vi "KHE - Main.vi"() -> ()   [LabVIEW 2016]
doc: "Use this template to build a producer/consumer design pattern with events to produce queue items. Use this design pattern instead of the User Interface Event Handler pattern for user interfaces when you want to execute code asynchronously in response to an event without slowing the user interface responsiveness."
uses:
  Hall Effect Library/Public/Controls/Resisitivity.ctl
  Hall Effect Library/Public/Controls/Magnets.ctl
  Hall Effect Library/Public/Controls/Ammeters.ctl
  Hall Effect Library/Public/Controls/I-Sources.ctl
  Hall Effect Library/Public/Controls/Switches.ctl
  Hall Effect Library/Public/Controls/Voltmeters.ctl
  <vilib>/Utility/miscctls.llb/LVPointTypeDef.ctl
  Hall Effect Library/Public/Communication/Decode Message Data (Status).vi
  Hall Effect Library/Public/Communication/Decode Message Data (New Data).vi
  Hall Effect Library/Public/Communication/Decode Message Data (Test End).vi
  Hall Effect Library/Hall Effect Library.lvlib
panel:
  in  "Front Panel Window Default Size":T1={"Horizontal"=980, "Vertical"=600}
  in  "cmdSaveData":bool
  in  "cmdClearData":bool
  out "Test Progress":u8(slide) scale=0.0..100.0
  in  "Instrument Locations":T2
  in  "Instruments":T8={"Magnet"=enum."Manual", "Ammeter"=enum."648X", "Current Source"=enum."622X", "Switch"=enum."3706A", "Voltmeter"=enum."2182A"}
  in  "Special Guard Parameters":T9={"Low to Earth"=enum."Off", "Inner Shield"=enum."Cable Guard"}
  out "Test In Progress":bool
  in  "cmdStop":bool
  in  "cmdStart":bool
  out "Status":string
  out "Programable Event":refnum<user-event>
  in  "Tab Control":T10(tab)
  in  "Test Type":T11
  in  "Test Identification":T12
  in  "Test Input Parameters":T14={"Current Level "=0.001, "Compliance Level"=1.0, "Soak Time"=0.0, "NPLC Voltmeter"=1.0, "Count Voltmeter"=1, "NPLC Ammeter"=1.0, "Count Ammeter"=1, "Sample Resistivity"=enum."Low", "Sample Thickness"=1.0, "Magnetic Flux"=0.57, "Units"=enum."T", "Sample Dimensions x"=1.0, "Sample Dimensions y"=1.0, "Sample Dimensions D1"=1.0, "Sample Dimensions D2"=1.0, "Sample Width Ws"=1.0, "Slot Number of 3765 Card"=1} {"Slot Number of 3765 Card" min=1 max=6 step=1; "NPLC Ammeter" min=0.01 max=10.0; "NPLC Voltmeter" min=0.01 max=10.0 format="%^#_6g"; "Count Ammeter" min=1 max=1024; "Count Voltmeter" min=1 max=1024; "Magnetic Flux" min=0.0; "Soak Time" min=0.0 format="%^#_6g"; "Sample Thickness" min=0.0; "Current Level" min=0.0 max=0.1 format="%^#_6e"; "Compliance Level" min=0.0 max=8.0 format="%^#_6g"}
  out "Test Date":string
  out "Hall Effect Results":T15 {"µH" format="%^#_6e"; "RHD" format="%^#_6e"; "RHC" format="%^#_6e"; "RHAvg" format="%^#_6e"; "n/p" format="%^#_6e"}
  out "Van Der Pauw Resistance Results":T16 {"PAvg" format="%^#_6e"; "PB" format="%^#_6e"; "PA" format="%^#_6e"; "QB" format="%^#_6e"; "QA" format="%^#_6e"; "fA" format="%^#_6e"; "fB" format="%^#_6e"}
  out "Hall Measurements":T17 {"V4" format="%^#_6e"; "V8" format="%^#_6e"; "V7" format="%^#_6e"; "V3" format="%^#_6e"; "V2" format="%^#_6e"; "V6" format="%^#_6e"; "V5" format="%^#_6e"; "V1" format="%^#_6e"}
  out "Van Der Pauw Measurements":T17 {"V7" format="%^#_6e"; "V8" format="%^#_6e"; "V6" format="%^#_6e"; "V5" format="%^#_6e"; "V4" format="%^#_6e"; "V3" format="%^#_6e"; "V2" format="%^#_6e"; "V1" format="%^#_6e"}
  out "Test Settings":T18={"Current Level"=0.0, "Compliance Level"=0.0, "Soak Time"=0.0, "NPLC Voltmeter"=1.0, "Count Voltmeter"=1, "NPLC Ammeter"=1.0, "Count Ammeter"=1, "Sample Resistivity"=enum."Low", "Sample Thickness"=0.0, "Magnetic Flux"=0.0, "Units"=enum."T", "Sample Dimensions x"=0.0, "Sample Dimension y"=0.0, "Sample Dimensions D1"=0.0, "Sample Dimensions D2"=0.0, "Sample Width Ws"=0.0, "Slot Number of 3765 Card"=0} {"NPLC Ammeter" min=0.01 max=10.0; "NPLC Voltmeter" min=0.01 max=10.0 format="%^#_6g"; "Count Ammeter" min=1 max=1024; "Count Voltmeter" min=1 max=1024; "Soak Time" format="%^#_6g"; "Compliance Level" format="%^#_6g"; "Current Level" format="%^#_6e"}
  out "Sample Name":string
  out "User Name":string
  out "8-Contact Sample Results":T19 {"uH" format="%^#_6e"; "RAVG" format="%^#_6e"; "PB" format="%^#_6e"; "PA" format="%^#_6e"; "Pavg" format="%^#_6e"}
  out "6-Contact Sample Results":T20 {"uH" format="%^#_6e"; "RH2" format="%^#_6e"; "RH1" format="%^#_6e"; "RAVG" format="%^#_6e"; "PB" format="%^#_6e"; "PA" format="%^#_6e"; "Pavg" format="%^#_6e"}
  out "8-Contact Sample Hall Voltage Measurements":cluster{"V1":dbl, "V2":dbl, "V3":dbl, "V4":dbl} {"V4" format="%^#_6e"; "V3" format="%^#_6e"; "V2" format="%^#_6e"; "V1" format="%^#_6e"}
  out "6-Contact Sample Hall Voltage Measurements":T21 {"V4" format="%^#_6e"; "V8" format="%^#_6e"; "V7" format="%^#_6e"; "V6" format="%^#_6e"; "V5" format="%^#_6e"; "V3" format="%^#_6e"; "V2" format="%^#_6e"; "V1" format="%^#_6e"}
  out "Bar Sample Results":T22 {"Hall Mobility" format="%^#_6e"; "n/p" format="%^#_6e"; "Resitivity" format="%^#_6e"}
  out "8-Contact Sample Resitivity Measurements":cluster{"V1":dbl, "V2":dbl, "V3":dbl, "V4":dbl} {"V4" format="%^#_6e"; "V3" format="%^#_6e"; "V2" format="%^#_6e"; "V1" format="%^#_6e"}
  out "6-Contact Sample Resitivity Measurements":cluster{"V1":dbl, "V2":dbl, "V3":dbl, "V4":dbl} {"V4" format="%^#_6e"; "V3" format="%^#_6e"; "V2" format="%^#_6e"; "V1" format="%^#_6e"}
  out "Bar Sample Measurements":T23 {"Hall Voltage" format="%^#_6e"; "Voltage Resistivity" format="%^#_6e"}
  in  "cmdBack":bool
  in  "cmdIndex":bool
  in  "Help Browser":refnum<k7>(container)
  # "Selecting Resistivity"
  # "Source Settings"
  # "A"
  # "V"
  # "s"
  # "Measure Settings"
  # "Ammeter"
  # "Voltmeter"
  # "Other Settings"
  # "cm"
  # "cm"
  # "cm"
  # "cm"
  # "cm"
  # "cm"
  # "Hall Coefficient"
  # "cm^3/C"
  # "cm^2/V s"
  # "cm^-3"
  # "cm^3/C"
  # "cm^3/C"
  # "Geometric Factor"
  # "Resistance Ratio"
  # "Resistivity"
  # "Ohm cm"
  # "Ohm cm"
  # "Ohm cm"
  # "Magnet"
  # "Pos"
  # "Volts"
  # "Neg"
  # "Polarity"
  # "Volts"
  # "A"
  # "V"
  # "s"
  # "NPLC"
  # "cm"
  # "Measure Count"
  # "cm"
  # "cm"
  # "cm"
  # "cm"
  # "cm"
  # "Resistivity"
  # "Hall Coefficient"
  # "Hall Mobility"
  # "PAvg"
  # "RH"
  # "µH"
  # "Ohm cm"
  # "cm^3/C"
  # "cm^2/V s"
  # "PA"
  # "Ohm cm"
  # "PB"
  # "Ohm cm"
  # "Resistivity"
  # "Hall Coefficient"
  # "Hall Mobility"
  # "PAvg"
  # "µH"
  # "RAvg"
  # "Ohm cm"
  # "cm^3/C"
  # "cm^2/V s"
  # "PA"
  # "RH1"
  # "Ohm cm"
  # "cm^3/C"
  # "PB"
  # "RH2"
  # "Ohm cm"
  # "cm^3/C"
  # "Magnet"
  # "V1"
  # "V2"
  # "Pos"
  # "Volts"
  # "Neg"
  # "Polarity"
  # "V3"
  # "V4"
  # "V1"
  # "V2"
  # "V5"
  # "V6"
  # "Magnet"
  # "Pos"
  # "Volts"
  # "Neg"
  # "Polarity"
  # "V3"
  # "V4"
  # "V7"
  # "V8"
  # "p"
  # "µH"
  # "Ohm cm"
  # "cm^-3"
  # "cm^2/V s"
  # "V1"
  # "V2"
  # "Current"
  # "Pos"
  # "Volts"
  # "Neg"
  # "Direction"
  # "V3"
  # "V4"
  # "V1"
  # "V2"
  # "Current"
  # "Pos"
  # "Volts"
  # "Neg"
  # "Direction"
  # "V3"
  # "V4"
  # "Vr"
  # "Vh"
  # "Volts"
  # "Volts"
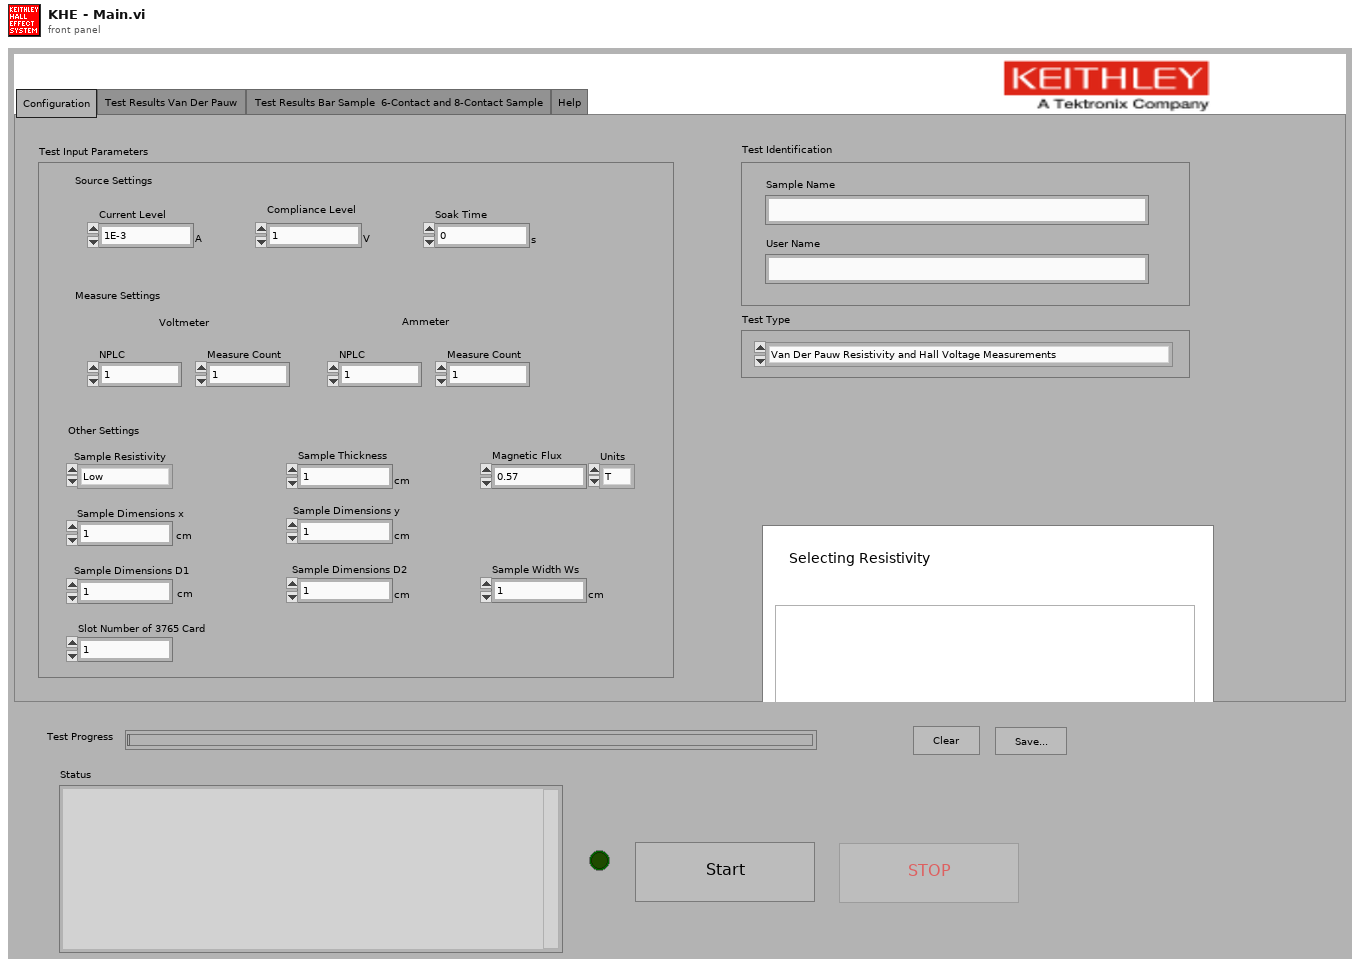
[diagram p1: front panel]
types:
  T1 = typedef "LVPointTypeDef.ctl" = cluster{"Horizontal":i16, "Vertical":i16}
  T2 = cluster{"Magnet Location":refnum<visa-resource-name>, "Ammeter Location":refnum<visa-resource-name>, "Current Source Location":refnum<visa-resource-name>, "Switch Location":refnum<visa-resource-name>, "Voltmeter Location":refnum<visa-resource-name>}
  T3 = typedef "Hall Effect Library.lvlib/Magnets.ctl" = enum16{"Manual"}
  T4 = typedef "Hall Effect Library.lvlib/Ammeters.ctl" = enum16{"None", "648X"}
  T5 = typedef "Hall Effect Library.lvlib/I-Sources.ctl" = enum16{"622X", "26XX"}
  T6 = typedef "Hall Effect Library.lvlib/Switches.ctl" = enum16{"3706A"}
  T7 = typedef "Hall Effect Library.lvlib/Voltmeters.ctl" = enum16{"2000", "2182A", "3706A"}
  T8 = cluster{"Magnet":T3, "Ammeter":T4, "Current Source":T5, "Switch":T6, "Voltmeter":T7}
  T9 = cluster{"Low to Earth":enum16{"On", "Off"}, "Inner Shield":enum16{"Output Lo ", "Cable Guard"}}
  T10 = enum32{"Configuration", "Test Results Van Der Pauw ", "Test Results Bar Sample  6-Contact and 8-Contact Sample ", "Help"}
  T11 = cluster{"Test Type":enum16{"Van Der Pauw Resistivity and Hall Voltage Measurements", "Bar Sample Resistivity and Hall Voltage Measurement", "6-Contact Sample Resistivity and Hall Voltage Measurement", "8-Contact Sample Resistivity and Hall Voltage Measurement"}}
  T12 = cluster{"Sample Name":string, "User Name":string}
  T13 = typedef "Hall Effect Library.lvlib/Resisitivity.ctl" = enum16{"Low", "High"}
  T14 = cluster{"Current Level ":dbl, "Compliance Level":dbl, "Soak Time":dbl, "NPLC Voltmeter":dbl, "Count Voltmeter":i32, "NPLC Ammeter":dbl, "Count Ammeter":i32, "Sample Resistivity":T13, "Sample Thickness":dbl, "Magnetic Flux":dbl, "Units":enum16{"Gs", "T"}, "Sample Dimensions x":dbl, "Sample Dimensions y":dbl, "Sample Dimensions D1":dbl, "Sample Dimensions D2":dbl, "Sample Width Ws":dbl, "Slot Number of 3765 Card":u32}
  T15 = cluster{"RHD":dbl, "RHC":dbl, "RHAvg":dbl, "µH":dbl, "n/p":dbl}
  T16 = cluster{"fA":dbl, "fB":dbl, "QA":dbl, "QB":dbl, "PAvg":dbl, "PA":dbl, "PB":dbl}
  T17 = cluster{"V1":dbl, "V2":dbl, "V3":dbl, "V4":dbl, "V5":dbl, "V6":dbl, "V7":dbl, "V8":dbl}
  T18 = cluster{"Current Level":dbl, "Compliance Level":dbl, "Soak Time":dbl, "NPLC Voltmeter":dbl, "Count Voltmeter":i32, "NPLC Ammeter":dbl, "Count Ammeter":i32, "Sample Resistivity":T13, "Sample Thickness":dbl, "Magnetic Flux":dbl, "Units":enum16{"Gs", "T"}, "Sample Dimensions x":dbl, "Sample Dimension y":dbl, "Sample Dimensions D1":dbl, "Sample Dimensions D2":dbl, "Sample Width Ws":dbl, "Slot Number of 3765 Card":u8}
  T19 = cluster{"Pavg":dbl, "PA":dbl, "PB":dbl, "RAVG":dbl, "uH":dbl}
  T20 = cluster{"Pavg":dbl, "PA":dbl, "PB":dbl, "RAVG":dbl, "RH1":dbl, "RH2":dbl, "uH":dbl}
  T21 = cluster{"V1":dbl, "V2":dbl, "V3":dbl, "V5":dbl, "V6":dbl, "V7":dbl, "V8":dbl, "V4":dbl}
  T22 = cluster{"Resitivity":dbl, "n/p":dbl, "Hall Mobility":dbl}
  T23 = cluster{"Voltage Resistivity":dbl, "Hall Voltage":dbl}
  T24 = cluster{"Test Identification":cluster{"Sample Name":string, "User Name":string}, "Test Input Parameters":cluster{"Current Level ":dbl, "Compliance Level":dbl, "Soak Time":dbl, "NPLC Voltmeter":dbl, "Count Voltmeter":i32, "NPLC Ammeter":dbl, "Count Ammeter":i32, "Sample Resistivity":T13, "Sample Thickness":dbl, "Magnetic Flux":dbl, "Units":enum16{"Gs", "T"}, "Sample Dimensions x":dbl, "Sample Dimensions y":dbl, "Sample Dimensions D1":dbl, "Sample Dimensions D2":dbl, "Sample Width Ws":dbl, "Slot Number of 3765 Card":u32}, "Test Type":cluster{"Test Type":enum16{"Van Der Pauw Resistivity and Hall Voltage Measurements", "Bar Sample Resistivity and Hall Voltage Measurement", "6-Contact Sample Resistivity and Hall Voltage Measurement", "8-Contact Sample Resistivity and Hall Voltage Measurement"}}}
  T25 = enum16{"open", "replace", "create", "open or create", "replace or create", "replace or create with confirmation"}
  T26 = enum32{"invalid app kind", "Development System", "Run Time System", "Student Edition", "Embedded LabVIEW", "Evaluation", "Custom"}
  T27 = typedef "LVAllMonitorsDisplayTypeDef.ctl" = cluster{"Bounds":cluster{"Left":i16, "Top":i16, "Right":i16, "Bottom":i16}, "Depth":i16}[]
  T28 = cluster{"Bounds":cluster{"Left":i16, "Top":i16, "Right":i16, "Bottom":i16}, "Depth":i16}
  T29 = cluster{"Left":i16, "Top":i16, "Right":i16, "Bottom":i16}
  T30 = typedef "LVRectTypeDef.ctl" = cluster{"Left":i16, "Top":i16, "Right":i16, "Bottom":i16}
  T31 = enum16{"Van Der Pauw Resistivity and Hall Voltage Measurements", "Bar Sample Resistivity and Hall Voltage Measurement", "6-Contact Sample Resistivity and Hall Voltage Measurement", "8-Contact Sample Resistivity and Hall Voltage Measurement"}
  T32 = typedef "Hall Effect Library.lvlib/Message Types.ctl" = enum16{"Status", "New Data", "Test End Normal", "Test End User Abort", "Test End Error"}
  T33 = typedef "Hall Effect Library.lvlib/Data Items.ctl" = enum16{"V1 Van Der Pauw", "V2 Van Der Pauw", "V3 Van Der Pauw", "V4 Van Der Pauw", "V5 Van Der Pauw", "V6 Van Der Pauw", "V7 Van Der Pauw", "V8 Van Der Pauw", "V1 Hall Effect", "V2 Hall Effect", "V3 Hall Effect", "V4 Hall Effect", "V5 Hall Effect", "V6  Hall Effect", "V7 Hall Effect", "V8 Hall Effect", "V1 Res Bar", "V1 Hall Bar", "V1 Res 6-Cot", "V2 Res 6-Cot", "V3 Res 6-Cot", "V4 Res 6-Cot", "V1 Hall 6-Cot", "V2 Hall 6-Cot", "V3 Hall 6-Cot", "V4 Hall 6-Cot", "V5 Hall 6-Cot", "V6 Hall 6-Cot", "V7 Hall 6-Cot", "V8 Hall 6-Cot", "V1 Res 8-Cot", "V2 Res 8-Cot", "V3 Res 8-Cot", "V4 Res 8-Cot", "V1 Hall 8-Cot", "V2 Hall 8-Cot", "V3 Hall 8-Cot", "V4 Hall 8-Cot", "Van Der Pauw Results", "Hall Effect Results", "Bar Sample Resistivity Results", "Bar Sample Hall Results", "6-Contact Resistivity Results", "6-Contact Hall Results", "8-Contact Resistivity Results", "8-Contact Hall Results"}
  T34 = cluster{"Van Der Pauw Voltages[0]":dbl, "Van Der Pauw Voltages[1]":dbl, "Van Der Pauw Voltages[2]":dbl, "Van Der Pauw Voltages[3]":dbl, "Van Der Pauw Voltages[4]":dbl, "Van Der Pauw Voltages[5]":dbl, "Van Der Pauw Voltages[6]":dbl, "Van Der Pauw Voltages[7]":dbl}
  T35 = cluster{"Hall Effect Voltages[0]":dbl, "Hall Effect Voltages[1]":dbl, "Hall Effect Voltages[2]":dbl, "Hall Effect Voltages[3]":dbl, "Hall Effect Voltages[4]":dbl, "Hall Effect Voltages[5]":dbl, "Hall Effect Voltages[6]":dbl, "Hall Effect Voltages[7]":dbl}
  T36 = cluster{"6-Contact Sample Resistivity Voltage[0]":dbl, "6-Contact Sample Resistivity Voltage[1]":dbl, "6-Contact Sample Resistivity Voltage[2]":dbl, "6-Contact Sample Resistivity Voltage[3]":dbl}
  T37 = cluster{"6-Contact Sample Hall Voltages[0]":dbl, "6-Contact Sample Hall Voltages[1]":dbl, "6-Contact Sample Hall Voltages[2]":dbl, "6-Contact Sample Hall Voltages[3]":dbl, "6-Contact Sample Hall Voltages[4]":dbl, "6-Contact Sample Hall Voltages[5]":dbl, "6-Contact Sample Hall Voltages[6]":dbl, "6-Contact Sample Hall Voltages[7]":dbl}
  T38 = cluster{"8-Contact Sample Resistivity Voltages[0]":dbl, "8-Contact Sample Resistivity Voltages[1]":dbl, "8-Contact Sample Resistivity Voltages[2]":dbl, "8-Contact Sample Resistivity Voltages[3]":dbl}
  T39 = cluster{"8-Contact Sample Hall Voltages[0]":dbl, "8-Contact Sample Hall Voltages[1]":dbl, "8-Contact Sample Hall Voltages[2]":dbl, "8-Contact Sample Hall Voltages[3]":dbl}
  T40 = cluster{"fA":dbl, "fB":dbl, "QA":dbl, "QB":dbl, "pAvg":dbl, "pA":dbl, "pB":dbl}
  T41 = cluster{"RHD":dbl, "RHC":dbl, "RHAvg":dbl, "uH":dbl, "n/p":dbl}
  T42 = cluster{"RAvg":dbl, "RH1":dbl, "RH2":dbl, "uH":dbl}
  T43 = typedef "Hall Effect Library.lvlib/Tests.ctl" = enum16{"Van Der Pauw", "Hall Effect", "Bar Sample Resistivity", "Bar Sample Hall ", "6-Contact Sample Resistivity", "6-Contact Sample Hall", "8-Contact Sample Resistivity", "8-Contact Sample Hall", ""}
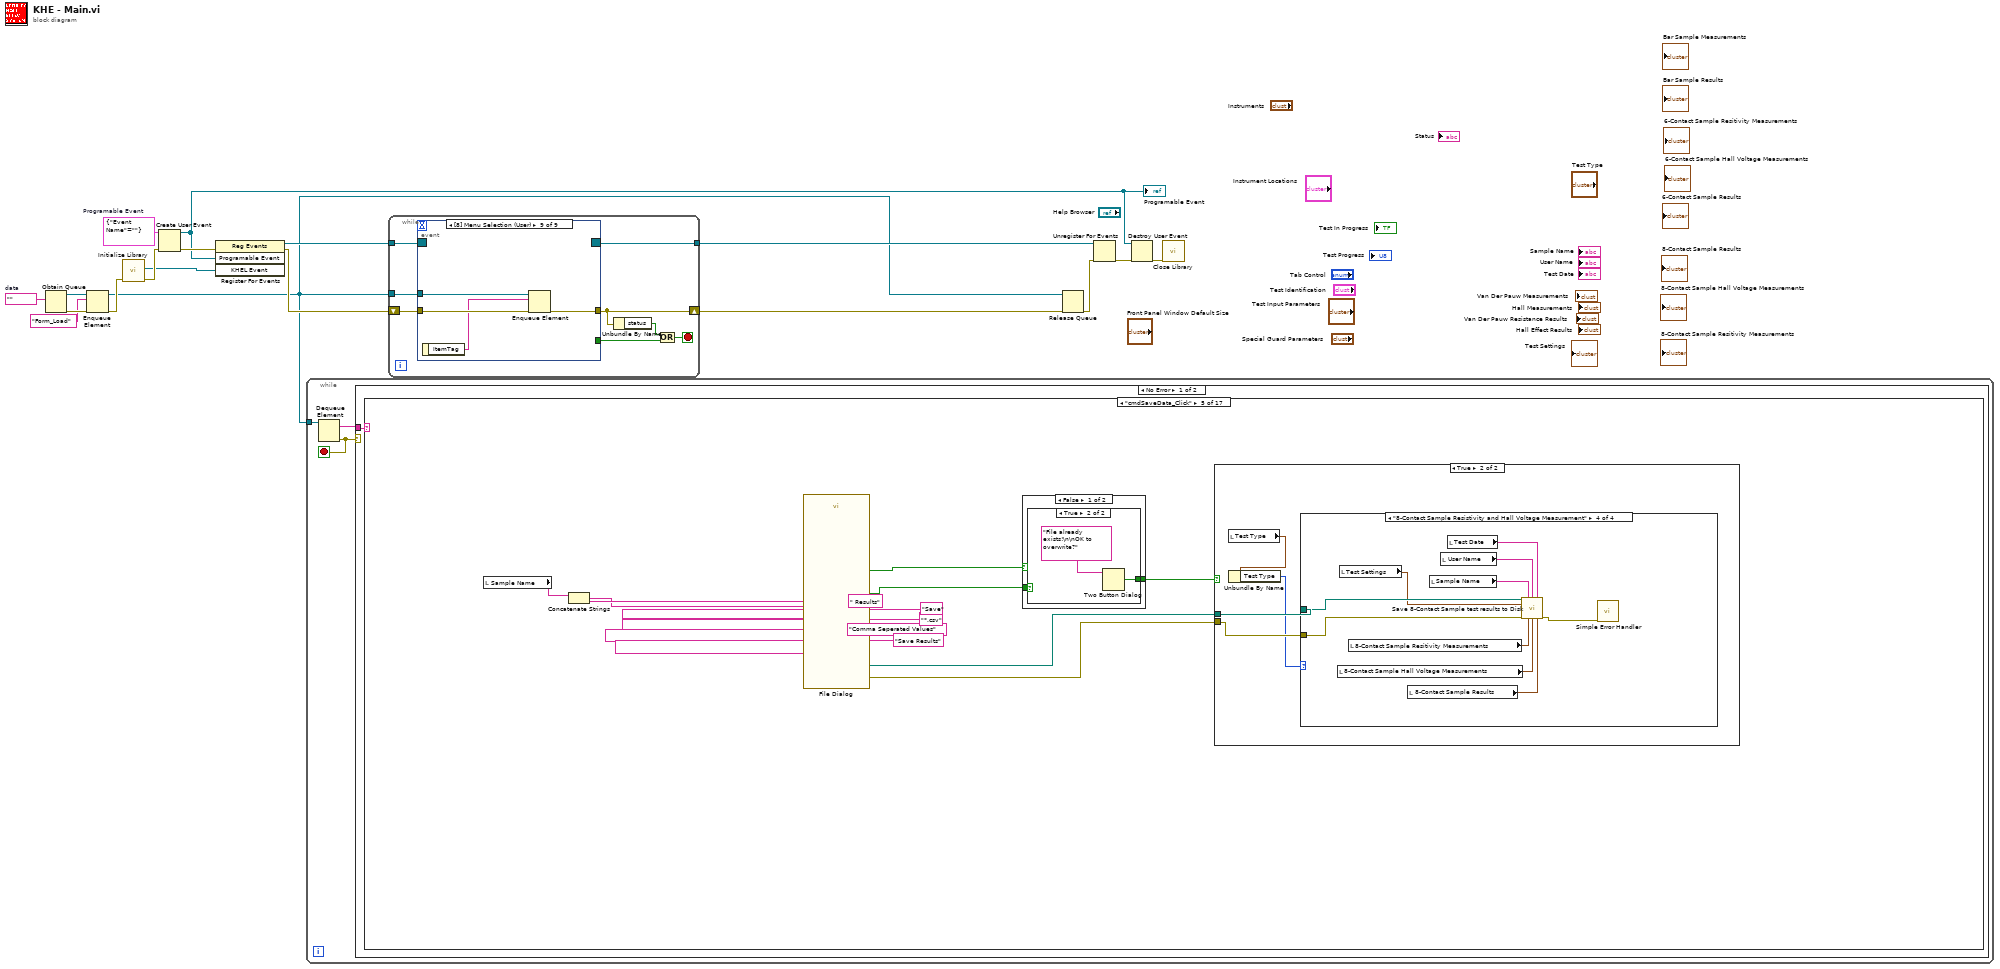
[diagram p0: block diagram]
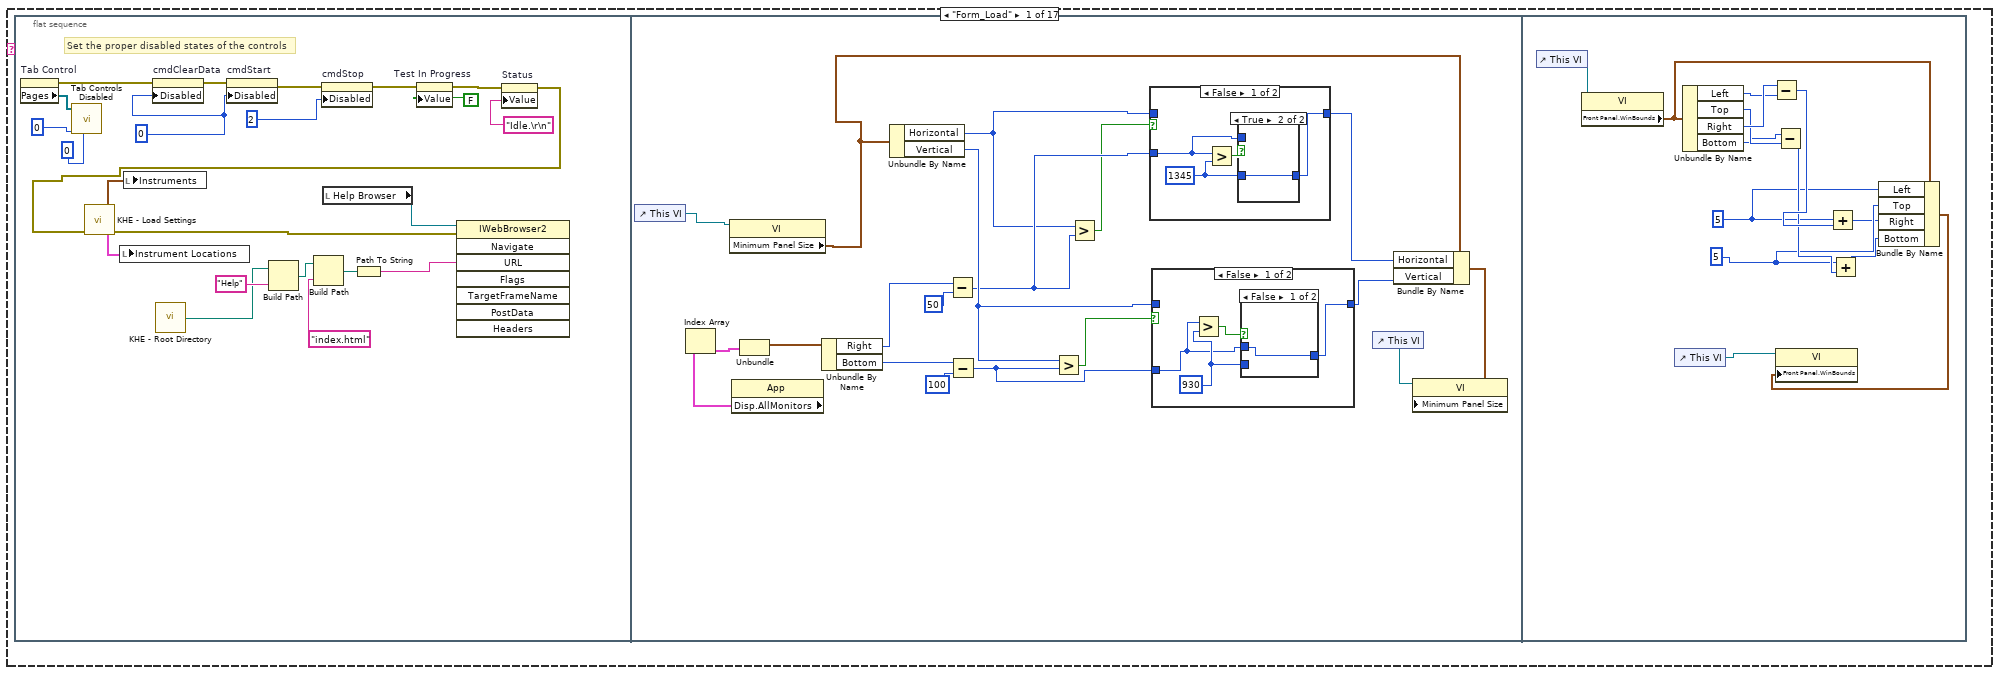
[diagram p2: hidden frame]
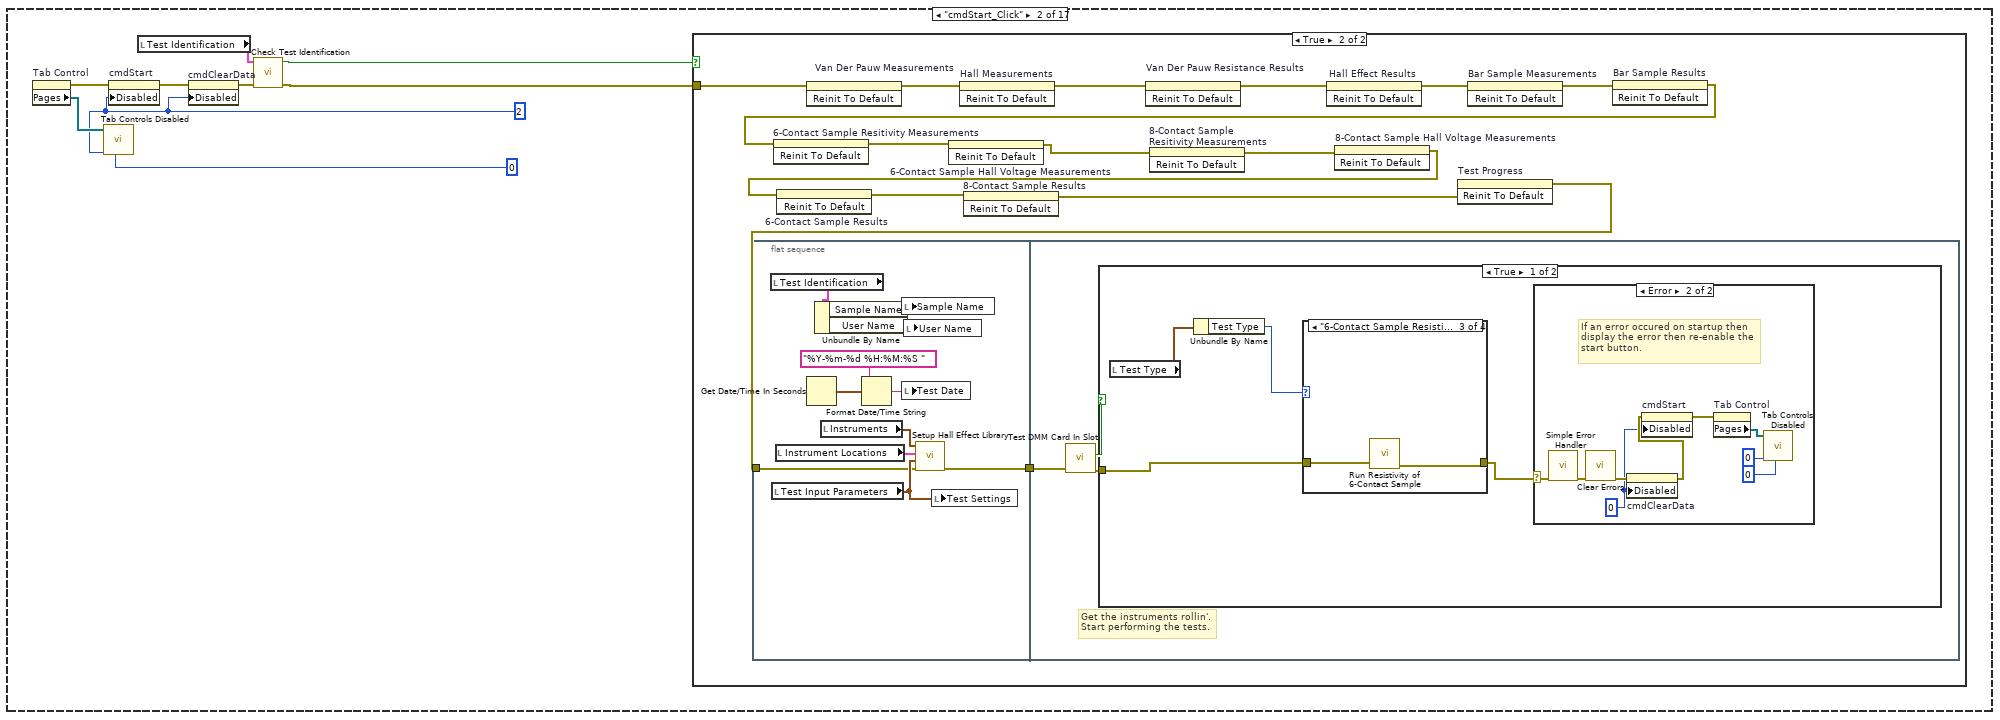
[diagram p7: hidden frame]
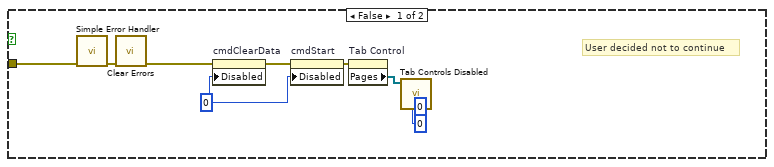
[diagram p8: hidden frame]
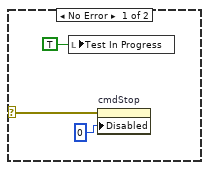
[diagram p9: hidden frame]
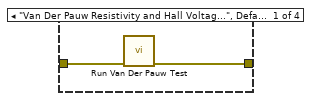
[diagram p10: hidden frame]
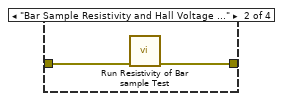
[diagram p11: hidden frame]
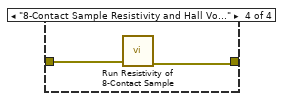
[diagram p12: hidden frame]
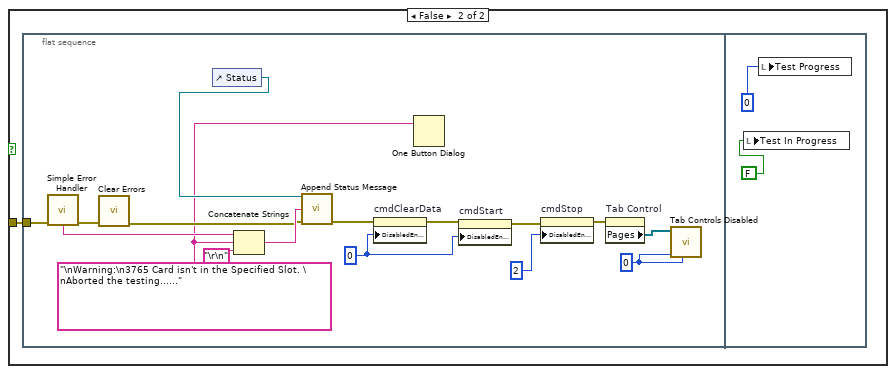
[diagram p13: hidden frame]
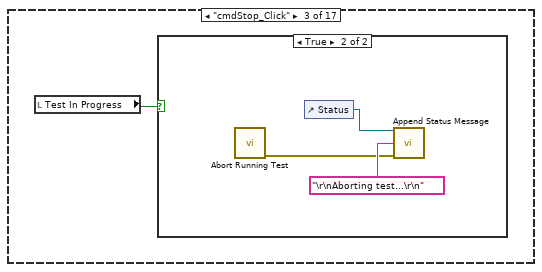
[diagram p14: hidden frame]
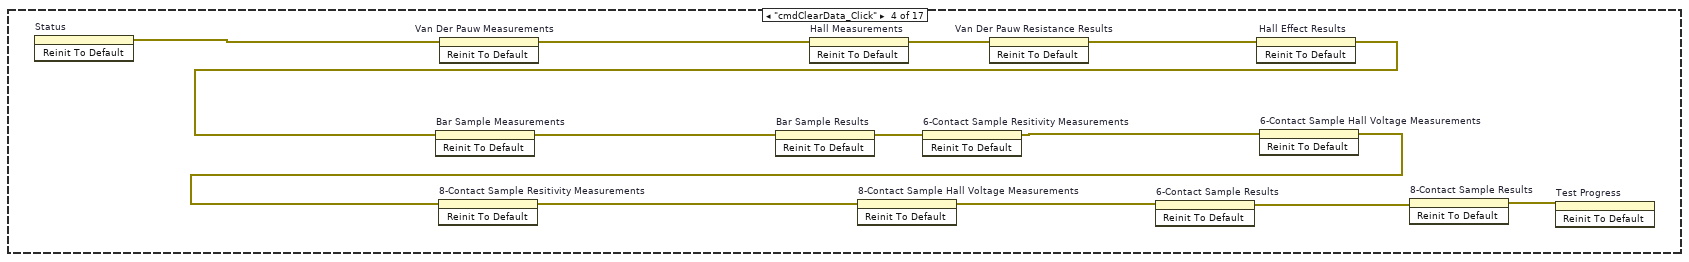
[diagram p16: hidden frame]
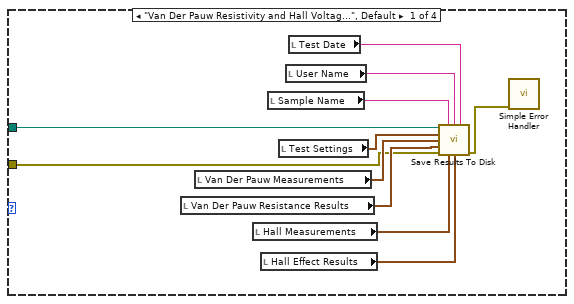
[diagram p18: hidden frame]
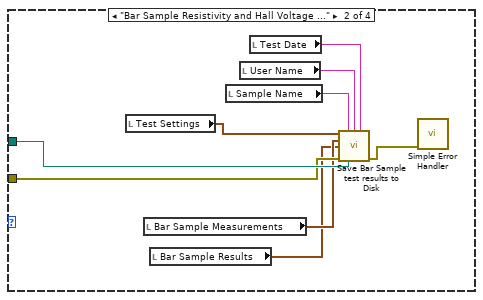
[diagram p19: hidden frame]
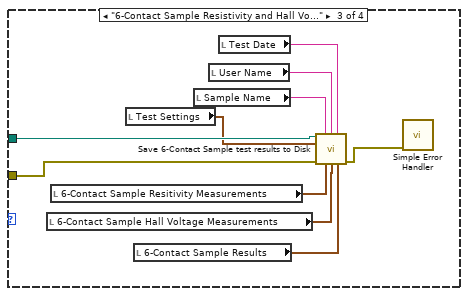
[diagram p20: hidden frame]
diagram:
  w16 = cluster{"Event Name":string} {"Event Name"=""}  # Programable Event
  w17 = ""  # data
  n1 = Obtain Queue(element data type=w17) -> (queue out=w9:refnum<queue>, error out=w8:errorcluster)  [unwired: 3 in, 2 out]
  n2 = Enqueue Element(queue=w9, element="Form_Load", error in (no error)=w8) -> (queue out=w2:refnum<queue>, error out=w6:errorcluster)  [unwired: 2 out]
  n3 = call "Initialize Library.vi"("error in (no error)"=w6) -> ("error out"=w5:errorcluster, "KHEL Event"=w3:refnum<user-event>)  [unwired: 9 out]
  n4 = Create User Event(user event datatype=w16, error in=w5) -> (user event=w4:refnum<user-event>, error out=w15:errorcluster)
  "Programable Event" <- w4
  n5 = register-events(error in=w15, w4, w3) -> (reference out=w10:refnum<event-registration>, error out=w14:errorcluster)  [unwired: 1 in]
  n6 = while {
    tunnel: w2 -> [w21]
    stop <- w20 stop-if-true
    n7 = Dequeue Element(queue=w21) -> (element=w19:string, error out=w20:errorcluster)  [unwired: 1 in, 3 out]
    n8 = case shown="No Error" w20 {
      tunnel: w19 -> [w22 _]
      frame No Error {
        n9 = case shown="\"cmdSaveData_Click\"" w22 {
          frame "Form_Load" {
            n10 = flat-sequence {
              frame #0 {
                w25 = u8 0 ("Disabled")
                # "Set the proper disabled states of the controls"
                n11 = property on="Tab Control" class="TabCtl (strict)"() -> (error out=w32:errorcluster, "Pages"=w44:refnum<vi>[])  [unwired: 2 in, 1 out]
                n12 = call "Tab Controls Disabled.vi"("Page"=0, "Disabled"=u8 0, "Tab Control Pages"=w44) -> ()  [unwired: 9 out]
                n13 = property on="cmdClearData" class="Bool"(error in=w32, "Disabled"=w25) -> (error out=w33:errorcluster)  [unwired: 1 in, 1 out]
                n14 = call "KHE - Root Directory.vi"() -> ("Project Root Directory"=w28:path)  [unwired: 1 out]
                n15 = property on="cmdStart" class="Bool"(error in=w33, "Disabled"=w25) -> (error out=w45:errorcluster)  [unwired: 1 in, 1 out]
                n16 = Build Path(base path=w28, name or relative path="Help") -> (appended path=w37:path)
                n17 = Build Path(base path=w37, name or relative path="index.html") -> (appended path=w35:path)
                n18 = property on="cmdStop" class="Bool"(error in=w45, "Disabled"=u8 2) -> (error out=w43:errorcluster)  [unwired: 1 in, 1 out]
                n19 = local read "Help Browser"() -> (w39:refnum<k7>)
                n20 = Path To String(path=w35) -> (string=w34:string)
                n21 = property on="Test In Progress" class="Bool (strict)"(error in=w43, "Value"=FALSE ("Test In Progress")) -> (error out=w41:errorcluster)  [unwired: 1 in, 1 out]
                n22 = property on="Status" class="Str"(error in=w41, "Value"="Idle.\r\n" ("Status")) -> (error out=w23:errorcluster)  [unwired: 1 in, 1 out]
                n23 = call "KHE - Load Settings.vi"("error in (no error)"=w23) -> ("error out"=w29:errorcluster, "Instrument Locations"=w31:T2, "Instruments"=w30:T8)  [unwired: 8 out]
                n24 = local write "Instrument Locations"(w31) -> ()
                n25 = local write "Instruments"(w30) -> ()
                n26 = invoke class="IWebBrowser2" method="Navigate"(reference=w39, error in=w29, "URL"=w34) -> ()  [unwired: 5 in, 8 out]
              }
              frame #1 {
                n27 = control-ref of="This VI"() -> (w46:refnum<vi>)
                n28 = property class="VI"(reference=w46) -> ("Minimum Panel Size"=w64:T1)  [unwired: 1 in, 2 out]
                n29 = property class="App"() -> ("Disp.AllMonitors"=w47:T27)  [unwired: 2 in, 2 out]
                n30 = Index Array(array=w47) -> (element=w48:T28)  [unwired: 1 in]
                n31 = Unbundle(w48) -> ("Bounds"=w49:T29)  [unwired: 1 out]
                n32 = Unbundle By Name(w49) -> ("Right"=w50:i16, "Bottom"=w52:i16)
                n33 = Unbundle By Name(w64) -> ("Horizontal"=w56:i16, "Vertical"=w58:i16)
                n34 = Subtract(x=w50, y=50) -> (x-y=w57:i32)
                n35 = Subtract(x=w52, y=100) -> (x-y=w59:i32)
                n36 = Greater?(x=w58, y=w59) -> (0:w55:bool)
                n37 = Greater?(x=w56, y=w57) -> (0:w54:bool)
                n38 = case shown="False" w54 {
                  tunnel: w56 -> [_ w78]
                  tunnel: w57 -> [w72 _]
                  tunnel: [w73 w78] -> w60
                  frame False {
                    w74 = 1345
                    n39 = Greater?(x=w72, y=w74) -> (0:w75:bool)
                    n40 = case shown="True" w75 {
                      tunnel: w74 -> [_ w77]
                      tunnel: [w76 w77] -> w73
                      tunnel: w72 -> [w76 _]
                      frame False {
                      }
                      frame True {
                      }
                    }
                  }
                  frame True {
                  }
                }
                n41 = case shown="False" w55 {
                  tunnel: w58 -> [_ w71]
                  tunnel: w59 -> [w65 _]
                  tunnel: [w66 w71] -> w61
                  frame False {
                    w67 = 930
                    n42 = Greater?(x=w65, y=w67) -> (0:w68:bool)
                    n43 = case shown="False" w68 {
                      tunnel: w67 -> [_ w70]
                      tunnel: [w69 w70] -> w66
                      tunnel: w65 -> [w69 _]
                      frame False {
                      }
                      frame True {
                      }
                    }
                  }
                  frame True {
                  }
                }
                n44 = control-ref of="This VI"() -> (w63:refnum<vi>)
                n45 = Bundle By Name(cluster=w64, "Horizontal"=w60, "Vertical"=w61) -> (w62:T1)
                n46 = property class="VI"(reference=w63, "Minimum Panel Size"=w62) -> ()  [unwired: 1 in, 2 out]
              }
              frame #2 {
                w84 = 5
                w85 = 5
                n47 = control-ref of="This VI"() -> (w92:refnum<vi>)
                n48 = property class="VI"(reference=w92) -> ("Front Panel.WinBounds"=w79:T30)  [unwired: 1 in, 2 out]
                n49 = control-ref of="This VI"() -> (w81:refnum<vi>)
                n50 = Unbundle By Name(w79) -> ("Left"=w90:i16, "Top"=w89:i16, "Right"=w91:i16, "Bottom"=w88:i16)
                n51 = Subtract(x=w91, y=w90) -> (x-y=w87:i16)
                n52 = Subtract(x=w88, y=w89) -> (x-y=w86:i16)
                n53 = Add(x=w85, y=w87) -> (x+y=w83:i32)
                n54 = Add(x=w84, y=w86) -> (x+y=w82:i32)
                n55 = Bundle By Name(cluster=w79, "Left"=w85, "Top"=w84, "Right"=w83, "Bottom"=w82) -> (w80:T30)
                n56 = property class="VI"(reference=w81, "Front Panel.WinBounds"=w80) -> ()  [unwired: 1 in, 2 out]
              }
            }
          }
          frame "cmdStart_Click" {
            w93 = u8 2 ("Disabled")
            n57 = property on="Tab Control" class="TabCtl (strict)"() -> (error out=w101:errorcluster, "Pages"=w100:refnum<vi>[])  [unwired: 2 in, 1 out]
            n58 = call "Tab Controls Disabled.vi"("Page"=0, "Disabled"=w93, "Tab Control Pages"=w100) -> ()  [unwired: 9 out]
            n59 = property on="cmdStart" class="Bool"(error in=w101, "Disabled"=w93) -> (error out=w95:errorcluster)  [unwired: 1 in, 1 out]
            n60 = local read "Test Identification"() -> (w98:T12)
            n61 = property on="cmdClearData" class="Bool"(error in=w95, "Disabled"=w93) -> (error out=w94:errorcluster)  [unwired: 1 in, 1 out]
            n62 = call "Check Test Identification.vi"("error in (no error)"=w94, "Test Identification"=w98) -> ("error out"=w97:errorcluster, "Continue?"=w96:bool)  [unwired: 8 out]
            n63 = case shown="True" w96 {
              tunnel: w97 -> [w105 w121]
              frame False {
                w102 = u8 0 ("Disabled")
                # "User decided not to continue"
                n64 = call <vilib>:"Simple Error Handler.vi"("error in (no error)"=w105) -> ("error out"=w110:errorcluster)  [unwired: 1 in, 7 out]
                n65 = call <vilib>:"Clear Errors.vi"("error in (no error)"=w110) -> ("error out"=w103:errorcluster)  [unwired: 1 in, 5 out]
                n66 = property on="cmdClearData" class="Bool"(error in=w103, "Disabled"=w102) -> (error out=w104:errorcluster)  [unwired: 1 in, 1 out]
                n67 = property on="cmdStart" class="Bool"(error in=w104, "Disabled"=w102) -> (error out=w108:errorcluster)  [unwired: 1 in, 1 out]
                n68 = property on="Tab Control" class="TabCtl (strict)"(error in=w108) -> ("Pages"=w109:refnum<vi>[])  [unwired: 1 in, 2 out]
                n69 = call "Tab Controls Disabled.vi"("Page"=0, "Disabled"=u8 0, "Tab Control Pages"=w109) -> ()  [unwired: 9 out]
              }
              frame True {
                n70 = flat-sequence {
                  tunnel: w122 -> [w127]
                  tunnel: [w126] -> w120
                  tunnel: w120 -> [w139]
                  frame #0 {
                    n71 = local read "Test Identification"() -> (w131:T12)
                    n72 = local read "Test Input Parameters"() -> (w130:T14)
                    n73 = local read "Instrument Locations"() -> (w128:T2)
                    n74 = Get Date/Time In Seconds() -> (seconds since 1Jan1904=w134:timestamp)
                    n75 = Unbundle By Name(w131) -> ("Sample Name"=w133:string, "User Name"=w132:string)
                    n76 = local read "Instruments"() -> (w129:T8)
                    n77 = Format Date/Time String(time format string (%c)="%Y-%m-%d %H:%M:%S ", seconds (now)=w134) -> (date/time string=w135:string)  [unwired: 1 out]
                    n78 = local write "Sample Name"(w133) -> ()
                    n79 = local write "Test Date"(w135) -> ()
                    n80 = local write "User Name"(w132) -> ()
                    n81 = call "Setup Hall Effect Library.vi"("error in (no error)"=w127, "Test Input Parameters"=w130, "Instrument Locations"=w128, "Instruments"=w129) -> ("error out"=w126:errorcluster)  [unwired: 7 out]
                    n82 = local write "Test Settings"(w130) -> ()
                  }
                  frame #1 {
                    # "Get the instruments rollin'.\nStart performing the tests."
                    n83 = call "Test DMM Card In Slot.vi"("error in (no error)"=w139) -> ("error out"=w137:errorcluster, "In Card Flag"=w138:bool)  [unwired: 9 in]
                    n84 = case shown="True" w138 {
                      tunnel: w137 -> [w143 w164]
                      frame True {
                        n85 = local read "Test Type"() -> (w141:T11)
                        n86 = Unbundle By Name(w141) -> ("Test Type"=w140:T31)
                        n87 = case shown="\"6-Contact Sample Resistivity and Hall Voltage Measurement\"" w140 {
                          tunnel: w143 -> [w156 w159 w161 w163]
                          tunnel: [w157 w158 w160 w162] -> w142
                          frame "Van Der Pauw Resistivity and Hall Voltage Measurements", Default {
                            n88 = call "Run Van Der Pauw Test.vi"("error in (no error)"=w156) -> ("error out"=w157:errorcluster)  [unwired: 10 out]
                          }
                          frame "Bar Sample Resistivity and Hall Voltage Measurement" {
                            n89 = call "Run Resistivity of Bar sample Test.vi"("error in (no error)"=w159) -> ("error out"=w158:errorcluster)  [unwired: 10 in]
                          }
                          frame "6-Contact Sample Resistivity and Hall Voltage Measurement" {
                            n90 = call "Run Resistivity of 6-Contact Sample.vi"("error in (no error)"=w161) -> ("error out"=w160:errorcluster)  [unwired: 10 in]
                          }
                          frame "8-Contact Sample Resistivity and Hall Voltage Measurement" {
                            n91 = call "Run Resistivity of 8-Contact Sample.vi"("error in (no error)"=w163) -> ("error out"=w162:errorcluster)  [unwired: 10 in]
                          }
                        }
                        n92 = case shown="Error" w142 {
                          selector: w142 -> [w145 w155]
                          frame No Error {
                            n93 = local write "Test In Progress"(TRUE ("Test In Progress")) -> ()
                            n94 = property on="cmdStop" class="Bool"(error in=w145, "Disabled"=u8 0) -> ()  [unwired: 1 in, 2 out]
                          }
                          frame Error {
                            w147 = u8 0 ("Disabled")
                            # "If an error occured on startup then\ndisplay the error then re-enable the\nstart button."
                            n95 = call <vilib>:"Simple Error Handler.vi"("error in (no error)"=w155) -> ("error out"=w154:errorcluster)  [unwired: 1 in, 7 out]
                            n96 = call <vilib>:"Clear Errors.vi"("error in (no error)"=w154) -> ("error out"=w149:errorcluster)  [unwired: 1 in, 5 out]
                            n97 = property on="cmdClearData" class="Bool"(error in=w149, "Disabled"=w147) -> (error out=w148:errorcluster)  [unwired: 1 in, 1 out]
                            n98 = property on="cmdStart" class="Bool"(error in=w148, "Disabled"=w147) -> (error out=w152:errorcluster)  [unwired: 1 in, 1 out]
                            n99 = property on="Tab Control" class="TabCtl (strict)"(error in=w152) -> ("Pages"=w153:refnum<vi>[])  [unwired: 1 in, 2 out]
                            n100 = call "Tab Controls Disabled.vi"("Page"=0, "Disabled"=u8 0, "Tab Control Pages"=w153) -> ()  [unwired: 9 out]
                          }
                        }
                      }
                      frame False {
                        n101 = flat-sequence {
                          tunnel: w164 -> [w179]
                          frame #0 {
                            w166 = 0
                            w170 = 0
                            w165 = "\nWarning:\n3765 Card isn't in the Specified Slot. \nAborted the testing......"
                            n102 = call <vilib>:"Simple Error Handler.vi"("error in (no error)"=w179) -> ("error out"=w175:errorcluster, "message"=w177:string)  [unwired: 1 in, 6 out]
                            n103 = call <vilib>:"Clear Errors.vi"("error in (no error)"=w175) -> ("error out"=w174:errorcluster)  [unwired: 1 in, 5 out]
                            n104 = control-ref of="Status"() -> (w180:refnum<vi>)
                            n105 = Concatenate Strings(w177, w165, "\r\n") -> (w176:string)
                            n106 = call "Append Status Message.vi"("Str Refnum"=w180, "Message"=w176, "error in (no error)"=w174) -> ("error out"=w173:errorcluster)  [unwired: 12 in]
                            n107 = property on="cmdClearData" class="Bool"(error in=w173, "DisabledEnum"=w170) -> (error out=w172:errorcluster)  [unwired: 1 in, 1 out]
                            n108 = One Button Dialog(message=w165) -> ()  [unwired: 1 in, 1 out]
                            n109 = property on="cmdStart" class="Bool"(error in=w172, "DisabledEnum"=w170) -> (error out=w171:errorcluster)  [unwired: 1 in, 1 out]
                            n110 = property on="cmdStop" class="Bool"(error in=w171, "DisabledEnum"=2) -> (error out=w168:errorcluster)  [unwired: 1 in, 1 out]
                            n111 = property on="Tab Control" class="TabCtl (strict)"(error in=w168) -> ("Pages"=w167:refnum<vi>[])  [unwired: 1 in, 2 out]
                            n112 = call "Tab Controls Disabled.vi"("Page"=w166, "Disabled"=w166, "Tab Control Pages"=w167) -> ()  [unwired: 9 in]
                          }
                          frame #1 {
                            n113 = local write "Test In Progress"(FALSE) -> ()
                            n114 = local write "Test Progress"(0) -> ()
                          }
                        }
                      }
                    }
                  }
                }
                n115 = invoke on="Van Der Pauw Measurements" class="Clust (strict)" method="Reinit To Default"(error in=w121) -> (error out=w125:errorcluster)  [unwired: 2 in, 2 out]
                n116 = invoke on="Hall Measurements" class="Clust (strict)" method="Reinit To Default"(error in=w125) -> (error out=w124:errorcluster)  [unwired: 2 in, 2 out]
                n117 = invoke on="Van Der Pauw Resistance Results" class="Clust (strict)" method="Reinit To Default"(error in=w124) -> (error out=w123:errorcluster)  [unwired: 2 in, 2 out]
                n118 = invoke on="Hall Effect Results" class="Clust (strict)" method="Reinit To Default"(error in=w123) -> (error out=w119:errorcluster)  [unwired: 2 in, 2 out]
                n119 = invoke on="Bar Sample Measurements" class="Clust (strict)" method="Reinit To Default"(error in=w119) -> (error out=w118:errorcluster)  [unwired: 2 in, 2 out]
                n120 = invoke on="Bar Sample Results" class="Clust (strict)" method="Reinit To Default"(error in=w118) -> (error out=w117:errorcluster)  [unwired: 2 in, 2 out]
                n121 = invoke on="6-Contact Sample Resitivity Measurements" class="Clust (strict)" method="Reinit To Default"(error in=w117) -> (error out=w116:errorcluster)  [unwired: 2 in, 2 out]
                n122 = invoke on="6-Contact Sample Hall Voltage Measurements" class="Clust (strict)" method="Reinit To Default"(error in=w116) -> (error out=w115:errorcluster)  [unwired: 2 in, 2 out]
                n123 = invoke on="8-Contact Sample Resitivity Measurements" class="Clust (strict)" method="Reinit To Default"(error in=w115) -> (error out=w114:errorcluster)  [unwired: 2 in, 2 out]
                n124 = invoke on="8-Contact Sample Hall Voltage Measurements" class="Clust (strict)" method="Reinit To Default"(error in=w114) -> (error out=w113:errorcluster)  [unwired: 2 in, 2 out]
                n125 = invoke on="6-Contact Sample Results" class="Clust (strict)" method="Reinit To Default"(error in=w113) -> (error out=w112:errorcluster)  [unwired: 2 in, 2 out]
                n126 = invoke on="8-Contact Sample Results" class="Clust (strict)" method="Reinit To Default"(error in=w112) -> (error out=w111:errorcluster)  [unwired: 2 in, 2 out]
                n127 = invoke on="Test Progress" class="Slide (strict)" method="Reinit To Default"(error in=w111) -> (error out=w122:errorcluster)  [unwired: 2 in, 2 out]
              }
            }
          }
          frame "cmdStop_Click" {
            n128 = local read "Test In Progress"() -> (w183:bool)
            n129 = case shown="True" w183 {
              frame False {
              }
              frame True {
                n130 = call "Abort Running Test.vi"() -> ("error out"=w184:errorcluster)  [unwired: 1 in, 10 out]
                n131 = control-ref of="Status"() -> (w186:refnum<vi>)
                n132 = call "Append Status Message.vi"("Str Refnum"=w186, "Message"="\r\nAborting test...\r\n", "error in (no error)"=w184) -> ()  [unwired: 13 out]
              }
            }
          }
          frame "cmdClearData_Click" {
            n133 = invoke on="Status" class="Str" method="Reinit To Default"() -> (error out=w187:errorcluster)  [unwired: 3 in, 2 out]
            n134 = invoke on="Van Der Pauw Measurements" class="Clust (strict)" method="Reinit To Default"(error in=w187) -> (error out=w199:errorcluster)  [unwired: 2 in, 2 out]
            n135 = invoke on="Hall Measurements" class="Clust (strict)" method="Reinit To Default"(error in=w199) -> (error out=w198:errorcluster)  [unwired: 2 in, 2 out]
            n136 = invoke on="Van Der Pauw Resistance Results" class="Clust (strict)" method="Reinit To Default"(error in=w198) -> (error out=w197:errorcluster)  [unwired: 2 in, 2 out]
            n137 = invoke on="Hall Effect Results" class="Clust (strict)" method="Reinit To Default"(error in=w197) -> (error out=w196:errorcluster)  [unwired: 2 in, 2 out]
            n138 = invoke on="Bar Sample Measurements" class="Clust (strict)" method="Reinit To Default"(error in=w196) -> (error out=w195:errorcluster)  [unwired: 2 in, 2 out]
            n139 = invoke on="Bar Sample Results" class="Clust (strict)" method="Reinit To Default"(error in=w195) -> (error out=w194:errorcluster)  [unwired: 2 in, 2 out]
            n140 = invoke on="6-Contact Sample Resitivity Measurements" class="Clust (strict)" method="Reinit To Default"(error in=w194) -> (error out=w193:errorcluster)  [unwired: 2 in, 2 out]
            n141 = invoke on="6-Contact Sample Hall Voltage Measurements" class="Clust (strict)" method="Reinit To Default"(error in=w193) -> (error out=w192:errorcluster)  [unwired: 2 in, 2 out]
            n142 = invoke on="8-Contact Sample Resitivity Measurements" class="Clust (strict)" method="Reinit To Default"(error in=w192) -> (error out=w191:errorcluster)  [unwired: 2 in, 2 out]
            n143 = invoke on="8-Contact Sample Hall Voltage Measurements" class="Clust (strict)" method="Reinit To Default"(error in=w191) -> (error out=w190:errorcluster)  [unwired: 2 in, 2 out]
            n144 = invoke on="6-Contact Sample Results" class="Clust (strict)" method="Reinit To Default"(error in=w190) -> (error out=w189:errorcluster)  [unwired: 2 in, 2 out]
            n145 = invoke on="8-Contact Sample Results" class="Clust (strict)" method="Reinit To Default"(error in=w189) -> (error out=w188:errorcluster)  [unwired: 2 in, 2 out]
            n146 = invoke on="Test Progress" class="Slide (strict)" method="Reinit To Default"(error in=w188) -> ()  [unwired: 2 in, 3 out]
          }
          frame "cmdSaveData_Click" {
            n147 = local read "Sample Name"() -> (w202:string)
            n148 = Concatenate Strings(w202, " Results" ("string")) -> (w200:string)
            n149 = call "File Dialog"("prompt"="Save Results", "button label"="Save", "default name"=w200, "pattern (all files)"="*.csv", "pattern label"="Comma Seperated Values") -> ("selected path"=w204:path, "exists"=w207:bool, "cancelled"=w208:bool, "error out"=w203:errorcluster)  [unwired: 2 in, 5 out]
            n150 = case shown="False" w208 {
              tunnel: w207 -> [w257 _]
              tunnel: [w256 FALSE ("T button?")] -> w206
              frame False {
                n151 = case shown="True" w257 {
                  tunnel: [TRUE ("T button?") w259] -> w256
                  frame False {
                  }
                  frame True {
                    n152 = Two Button Dialog(message="File already exists!\n\nOK to overwrite?") -> (T button?=w259:bool)  [unwired: 2 out]
                  }
                }
              }
              frame True {
              }
            }
            n153 = case shown="True" w206 {
              tunnel: w204 -> [_ w215]
              tunnel: w203 -> [_ w214]
              frame False {
              }
              frame True {
                n154 = local read "Test Type"() -> (w213:T11)
                n155 = Unbundle By Name(w213) -> ("Test Type"=w212:T31)
                n156 = case shown="\"8-Contact Sample Resistivity and Hall Voltage Measurement\"" w212 {
                  tunnel: w215 -> [w217 w232 w245 w254]
                  tunnel: w214 -> [w216 w231 w244 w253]
                  frame "Van Der Pauw Resistivity and Hall Voltage Measurements", Default {
                    n157 = local read "Van Der Pauw Resistance Results"() -> (w220:T16)
                    n158 = local read "Van Der Pauw Measurements"() -> (w221:T17)
                    n159 = local read "Hall Measurements"() -> (w219:T17)
                    n160 = local read "Hall Effect Results"() -> (w218:T15)
                    n161 = local read "Sample Name"() -> (w223:string)
                    n162 = local read "Test Settings"() -> (w222:T18)
                    n163 = local read "User Name"() -> (w224:string)
                    n164 = local read "Test Date"() -> (w225:string)
                    n165 = call "Save Results To Disk.vi"("Save To Path"=w217, "Sample Name"=w223, "User Name"=w224, "Test Date"=w225, "Test Settings"=w222, "Van Der Pauw Measurements"=w221, "Van Der Pauw Resistance Results"=w220, "error in (no error)"=w216, "Hall Measurements"=w219, "Hall Effect Results"=w218) -> ("error out"=w226:errorcluster)  [unwired: 5 out]
                    n166 = call <vilib>:"Simple Error Handler.vi"("error in (no error)"=w226) -> ()  [unwired: 1 in, 8 out]
                  }
                  frame "Bar Sample Resistivity and Hall Voltage Measurement" {
                    n167 = local read "Test Settings"() -> (w227:T18)
                    n168 = local read "Bar Sample Measurements"() -> (w230:T23)
                    n169 = local read "Bar Sample Results"() -> (w229:T22)
                    n170 = local read "Sample Name"() -> (w233:string)
                    n171 = local read "User Name"() -> (w234:string)
                    n172 = local read "Test Date"() -> (w235:string)
                    n173 = call "Save Bar Sample test results to Disk.vi"("Test Settings"=w227, "Sample Name"=w233, "User Name"=w234, "Test Date"=w235, "Bar Sample Measurements"=w230, "Bar Sample Results"=w229, "error in (no error)"=w231, "Save To Path"=w232) -> ("error out"=w228:errorcluster)  [unwired: 7 in]
                    n174 = call <vilib>:"Simple Error Handler.vi"("error in (no error)"=w228) -> ()  [unwired: 1 in, 8 out]
                  }
                  frame "6-Contact Sample Resistivity and Hall Voltage Measurement" {
                    n175 = local read "6-Contact Sample Hall Voltage Measurements"() -> (w238:T21)
                    n176 = local read "6-Contact Sample Resitivity Measurements"() -> (w239:cluster{"V1":dbl, "V2":dbl, "V3":dbl, "V4":dbl})
                    n177 = local read "Test Settings"() -> (w240:T18)
                    n178 = local read "6-Contact Sample Results"() -> (w237:T20)
                    n179 = local read "Sample Name"() -> (w241:string)
                    n180 = local read "User Name"() -> (w242:string)
                    n181 = local read "Test Date"() -> (w243:string)
                    n182 = call "Save 6-Contact Sample test results to Disk.vi"("Save To Path"=w245, "Sample Name"=w241, "User Name"=w242, "Test Date"=w243, "Test Settings"=w240, "error in (no error)"=w244, "6-Contact Sample Resitivity Measurements"=w239, "6-Contact Sample Hall Voltage Measurements"=w238, "6-Contact Sample Results"=w237) -> ("error out"=w236:errorcluster)  [unwired: 6 in]
                    n183 = call <vilib>:"Simple Error Handler.vi"("error in (no error)"=w236) -> ()  [unwired: 1 in, 8 out]
                  }
                  frame "8-Contact Sample Resistivity and Hall Voltage Measurement" {
                    n184 = local read "8-Contact Sample Hall Voltage Measurements"() -> (w247:cluster{"V1":dbl, "V2":dbl, "V3":dbl, "V4":dbl})
                    n185 = local read "Test Settings"() -> (w249:T18)
                    n186 = local read "8-Contact Sample Resitivity Measurements"() -> (w248:cluster{"V1":dbl, "V2":dbl, "V3":dbl, "V4":dbl})
                    n187 = local read "8-Contact Sample Results"() -> (w246:T19)
                    n188 = local read "Sample Name"() -> (w250:string)
                    n189 = local read "User Name"() -> (w251:string)
                    n190 = local read "Test Date"() -> (w252:string)
                    n191 = call "Save 8-Contact Sample test results to Disk.vi"("Save To Path"=w254, "Sample Name"=w250, "User Name"=w251, "Test Date"=w252, "Test Settings"=w249, "error in (no error)"=w253, "8-Contact Sample Resitivity Measurements"=w248, "8-Contact Sample Hall Voltage Measurements"=w247, "8-Contact Sample Results"=w246) -> ("error out"=w255:errorcluster)  [unwired: 6 in]
                    n192 = call <vilib>:"Simple Error Handler.vi"("error in (no error)"=w255) -> ()  [unwired: 1 in, 8 out]
                  }
                }
              }
            }
          }
          frame "cmdIndex_Click" {
            n193 = call "KHE - Root Directory.vi"() -> ("Project Root Directory"=w263:path)  [unwired: 1 out]
            n194 = Build Path(base path=w263, name or relative path="Help") -> (appended path=w266:path)
            n195 = local read "Help Browser"() -> (w264:refnum<k7>)
            n196 = Build Path(base path=w266, name or relative path="index.html") -> (appended path=w268:path)
            n197 = Path To String(path=w268) -> (string=w262:string)
            n198 = invoke class="IWebBrowser2" method="Navigate"(reference=w264, "URL"=w262) -> ()  [unwired: 6 in, 8 out]
          }
          frame "cmdBack_Click" {
            n199 = local read "Help Browser"() -> (w270:refnum<k7>)
            n200 = property class="IWebBrowser2"(reference=w270) -> ("LocationName"=w269:string)  [unwired: 1 in, 2 out]
            n201 = Equal?(x=w269, y="index.html") -> (x = y?=w271:bool)
            n202 = case shown="True" w271 {
              tunnel: w270 -> [w273 _]
              frame False {
                n203 = invoke class="IWebBrowser2" method="GoBack"(reference=w273) -> ()  [unwired: 2 in, 3 out]
              }
              frame True {
              }
            }
          }
          frame "cmdClose_Click" {
            n204 = local read "Test In Progress"() -> (w275:bool)
            n205 = case shown="True" w275 {
              selector: w275 -> [w282 _]
              tunnel: [w282 w283] -> w274
              frame False {
              }
              frame True {
                n206 = Two Button Dialog(message="Test is still in progress.\n\nAre you sure you\nwant to quit?", 1:"No" ("F button name (\"Cancel\")"), 2:"Yes" ("T button name (\"OK\")")) -> (T button?=w283:bool)
              }
            }
            n207 = case shown="True" w274 {
              frame False {
                n208 = local read "Programable Event"() -> (w276:refnum<user-event>)
                n209 = Generate User Event(user event=w276, event data cluster=cluster{string} {"QUIT"} ("event data")) -> ()  [unwired: 2 in, 2 out]
              }
              frame True {
                n210 = call "Abort Running Test.vi"() -> ("error out"=w279:errorcluster)  [unwired: 1 in, 10 out]
                n211 = call "Close Library.vi"("error in (no error)"=w279) -> ("error out"=w278:errorcluster)  [unwired: 10 out]
                n212 = local read "Programable Event"() -> (w280:refnum<user-event>)
                n213 = Generate User Event(user event=w280, event data cluster=cluster{string} {"QUIT"} ("event data"), error in=w278) -> ()  [unwired: 1 in, 2 out]
              }
            }
          }
          frame "KHEL_EVENT" {
            n214 = call "Get Message.vi"() -> ("Message Type"=w287:T32, "Data"=w288:variant, "error out"=w289:errorcluster)  [unwired: 1 in, 12 out]
            n215 = case shown="\"Status\", Default" w287 {
              tunnel: w288 -> [w292 w300 w392 w469]
              tunnel: w289 -> [w293 w302 w393 w470]
              frame "Status", Default {
                n216 = local read "Test Progress"() -> (w296:u8)
                n217 = call-poly "Decode Message Data.vi"("Message Data"=w292, "error in"=w293) -> ("Decoded Data"=w291:string, "error out"=w290:errorcluster)  [unwired: 12 out]
                n218 = control-ref of="Status"() -> (w298:refnum<vi>)
                n219 = Add(x=w296, y=u8 2) -> (x+y=w295:u8)
                n220 = call "Append Status Message.vi"("Str Refnum"=w298, "Message"=w291, "error in (no error)"=w290) -> ("error out"=w297:errorcluster)  [unwired: 12 out]
                n221 = local write "Test Progress"(w295) -> ()
                n222 = call <vilib>:"Simple Error Handler.vi"("error in (no error)"=w297) -> ()  [unwired: 1 in, 8 out]
              }
              frame "New Data" {
                # "New data is available.  See what it is then place it into the results."
                n223 = call-poly "Decode Message Data.vi"("Message Data"=w300, "error in"=w302) -> ("Decoded Data"=w299:T33, "error out"=w301:errorcluster)  [unwired: 12 out]
                n224 = case shown="\"V1 Hall Effect\"..\"V8 Hall Effect\"" w299 {
                  tunnel: w301 -> [w305 w308 w315 w324 w327 w330 w333 w336 w338 w340 w345 w353 w360 w372 w379 w389]
                  tunnel: [w305 w308 w315 w324 w327 w330 w333 w336 w338 w340 w345 w353 w360 w372 w379 w389] -> w303
                  frame "V1 Van Der Pauw".."V8 Van Der Pauw", Default {
                    n225 = call "Recall Van Der Pauw Voltages.vi"() -> ("Van Der Pauw Voltages"=w304:dbl[])  [unwired: 11 out]
                    n226 = Array To Cluster(array=w304) -> (cluster=w306:T34)
                    n227 = local write "Van Der Pauw Measurements"(w306) -> ()
                  }
                  frame "V1 Hall Effect".."V8 Hall Effect" {
                    n228 = call "Recall Hall Effect Voltages.vi"() -> ("Hall Effect Voltages"=w307:dbl[])  [unwired: 11 out]
                    n229 = Array To Cluster(array=w307) -> (cluster=w309:T35)
                    n230 = local write "Hall Measurements"(w309) -> ()
                  }
                  frame "V1 Res Bar" {
                    n231 = call "Recall Bar Sample Resistivity Voltages.vi"() -> ("Bar  Sample Resistivity Voltages"=w313:dbl[])  [unwired: 11 in]
                    n232 = Index Array(array=w313, index=0) -> (element=w311:dbl)
                    n233 = Bundle By Name(cluster=T23 {"Voltage Resistivity"=0.0, "Hall Voltage"=0.0} ("Bar Sample Measurements"), "Voltage Resistivity"=w311) -> (w310:T23)
                    n234 = local write "Bar Sample Measurements"(w310) -> ()
                  }
                  frame "V1 Hall Bar" {
                    n235 = call "Recall Bar Sample Hall Voltages.vi"() -> ("Bar Sample Hall Voltage"=w323:dbl[])  [unwired: 11 in]
                    n236 = call "Recall Bar Sample Resistivity Voltages.vi"() -> ("Bar  Sample Resistivity Voltages"=w318:dbl[])  [unwired: 11 in]
                    n237 = Index Array(array=w318, index=0) -> (element=w316:dbl)
                    n238 = Index Array(array=w323, index=0) -> (element=w320:dbl)
                    n239 = Bundle By Name(cluster=T23 {"Voltage Resistivity"=0.0, "Hall Voltage"=0.0} ("Bar Sample Measurements"), "Hall Voltage"=w320, "Voltage Resistivity"=w316) -> (w319:T23)
                    n240 = local write "Bar Sample Measurements"(w319) -> ()
                  }
                  frame "V1 Res 6-Cot".."V4 Res 6-Cot" {
                    n241 = call "Recall 6-Contact Sample Resistivity Voltages.vi"() -> ("6-Contact Sample Resistivity Voltage"=w326:dbl[])  [unwired: 11 in]
                    n242 = Array To Cluster(array=w326) -> (cluster=w325:T36)
                    n243 = local write "6-Contact Sample Resitivity Measurements"(w325) -> ()
                  }
                  frame "V1 Hall 6-Cot".."V8 Hall 6-Cot" {
                    n244 = call "Recall 6-Contact Sample Hall Voltages.vi"() -> ("6-Contact Sample Hall Voltages"=w329:dbl[])  [unwired: 11 in]
                    n245 = Array To Cluster(array=w329) -> (cluster=w328:T37)
                    n246 = local write "6-Contact Sample Hall Voltage Measurements"(w328) -> ()
                  }
                  frame "V1 Res 8-Cot".."V4 Res 8-Cot" {
                    n247 = call "Recall 8-Contact Sample Resistivity Voltages.vi"() -> ("8-Contact Sample Resistivity Voltages"=w332:dbl[])  [unwired: 11 in]
                    n248 = Array To Cluster(array=w332) -> (cluster=w331:T38)
                    n249 = local write "8-Contact Sample Resitivity Measurements"(w331) -> ()
                  }
                  frame "V1 Hall 8-Cot".."V4 Hall 8-Cot" {
                    n250 = call "Recall 8-Contact Sample Hall Voltages.vi"() -> ("8-Contact Sample Hall Voltages"=w335:dbl[])  [unwired: 11 in]
                    n251 = Array To Cluster(array=w335) -> (cluster=w334:T39)
                    n252 = local write "8-Contact Sample Hall Voltage Measurements"(w334) -> ()
                  }
                  frame "Van Der Pauw Results" {
                    n253 = call "Recall Van Der Pauw Results.vi"() -> ("Van Der Pauw Results"=w337:T40)  [unwired: 11 out]
                    n254 = local write "Van Der Pauw Resistance Results"(w337) -> ()
                  }
                  frame "Hall Effect Results" {
                    n255 = call "Recall Hall Effect Results.vi"() -> ("Hall Effect Results"=w339:T41)  [unwired: 11 out]
                    n256 = local write "Hall Effect Results"(w339) -> ()
                  }
                  frame "Bar Sample Resistivity Results" {
                    n257 = call "Recall Bar Sample Resistivity Results.vi"() -> ("Bar Sample Resistivity Results"=w344:cluster{"p":dbl})  [unwired: 11 in]
                    n258 = Unbundle By Name(w344) -> ("p"=w343:dbl)
                    n259 = Bundle By Name(cluster=T22 {"Resitivity"=0.0, "n/p"=0.0, "Hall Mobility"=0.0} ("Bar Sample Results"), "Resitivity"=w343) -> (w341:T22)
                    n260 = local write "Bar Sample Results"(w341) -> ()
                  }
                  frame "Bar Sample Hall Results" {
                    n261 = call "Recall Bar Sample Resistivity Results.vi"() -> ("Bar Sample Resistivity Results"=w349:cluster{"p":dbl})  [unwired: 11 in]
                    n262 = call "Recall Bar Sample Hall Results.vi"() -> ("Bar Sample Hall Results"=w352:cluster{"n/p":dbl, "uH":dbl})  [unwired: 11 in]
                    n263 = Unbundle By Name(w352) -> ("n/p"=w347:dbl, "uH"=w346:dbl)
                    n264 = Unbundle By Name(w349) -> ("p"=w348:dbl)
                    n265 = Bundle By Name(cluster=T22 {"Resitivity"=0.0, "n/p"=0.0, "Hall Mobility"=0.0} ("Bar Sample Results"), "Resitivity"=w348, "n/p"=w347, "Hall Mobility"=w346) -> (w350:T22)
                    n266 = local write "Bar Sample Results"(w350) -> ()
                  }
                  frame "6-Contact Resistivity Results" {
                    n267 = call "Recall 6-Contact Sample Resistivity Results.vi"() -> ("6-Contact Sample Resistivity Results"=w359:cluster{"PAvg":dbl, "PA":dbl, "PB":dbl})  [unwired: 11 in]
                    n268 = Unbundle By Name(w359) -> ("PAvg"=w357:dbl, "PA"=w356:dbl, "PB"=w355:dbl)
                    n269 = Bundle By Name(cluster=T20 {"Pavg"=0.0, "PA"=0.0, "PB"=0.0, "RAVG"=0.0, "RH1"=0.0, "RH2"=0.0, "uH"=0.0} ("6-Contact Sample Results"), "Pavg"=w357, "PA"=w356, "PB"=w355) -> (w354:T20)
                    n270 = local write "6-Contact Sample Results"(w354) -> ()
                  }
                  frame "6-Contact Hall Results" {
                    n271 = call "Recall 6-Contact Sample Resistivity Results.vi"() -> ("6-Contact Sample Resistivity Results"=w364:cluster{"PAvg":dbl, "PA":dbl, "PB":dbl})  [unwired: 11 in]
                    n272 = call "Recall 6-Contact Sample Hall Results.vi"() -> ("6-Contact Sample Hall Results"=w371:T42)  [unwired: 11 in]
                    n273 = Unbundle By Name(w364) -> ("PAvg"=w363:dbl, "PA"=w362:dbl, "PB"=w361:dbl)
                    n274 = Unbundle By Name(w371) -> ("RAvg"=w369:dbl, "RH1"=w368:dbl, "RH2"=w367:dbl, "uH"=w366:dbl)
                    n275 = Bundle By Name(cluster=T20 {"Pavg"=0.0, "PA"=0.0, "PB"=0.0, "RAVG"=0.0, "RH1"=0.0, "RH2"=0.0, "uH"=0.0} ("6-Contact Sample Results"), "RAVG"=w369, "RH1"=w368, "RH2"=w367, "uH"=w366, "Pavg"=w363, "PA"=w362, "PB"=w361) -> (w365:T20)
                    n276 = local write "6-Contact Sample Results"(w365) -> ()
                  }
                  frame "8-Contact Resistivity Results" {
                    n277 = call "Recall 8-Contact Sample Resistivity Results.vi"() -> ("8-Contact Sample Resistivity Results"=w378:cluster{"PAvg":dbl, "PA":dbl, "PB":dbl})  [unwired: 11 in]
                    n278 = Unbundle By Name(w378) -> ("PAvg"=w376:dbl, "PA"=w375:dbl, "PB"=w374:dbl)
                    n279 = Bundle By Name(cluster=T19 {"Pavg"=0.0, "PA"=0.0, "PB"=0.0, "RAVG"=0.0, "uH"=0.0} ("8-Contact Sample Results"), "Pavg"=w376, "PA"=w375, "PB"=w374) -> (w373:T19)
                    n280 = local write "8-Contact Sample Results"(w373) -> ()
                  }
                  frame "8-Contact Hall Results" {
                    n281 = call "Recall 8-Contact Sample Hall Results.vi"() -> ("8-Contact Sample Hall Results"=w388:cluster{"RH":dbl, "uH":dbl})  [unwired: 11 in]
                    n282 = call "Recall 8-Contact Sample Resistivity Results.vi"() -> ("8-Contact Sample Resistivity Results"=w383:cluster{"PAvg":dbl, "PA":dbl, "PB":dbl})  [unwired: 11 in]
                    n283 = Unbundle By Name(w383) -> ("PAvg"=w382:dbl, "PA"=w381:dbl, "PB"=w380:dbl)
                    n284 = Unbundle By Name(w388) -> ("RH"=w386:dbl, "uH"=w385:dbl)
                    n285 = Bundle By Name(cluster=T19 {"Pavg"=0.0, "PA"=0.0, "PB"=0.0, "RAVG"=0.0, "uH"=0.0} ("8-Contact Sample Results"), "RAVG"=w386, "uH"=w385, "Pavg"=w382, "PA"=w381, "PB"=w380) -> (w384:T19)
                    n286 = local write "8-Contact Sample Results"(w384) -> ()
                  }
                }
                n287 = call <vilib>:"Simple Error Handler.vi"("error in (no error)"=w303) -> ()  [unwired: 1 in, 8 out]
              }
              frame "Test End Normal" {
                n288 = call-poly "Decode Message Data.vi"("Message Data"=w392, "error in"=w393) -> ("Test"=w390:T43, "error out"=w391:errorcluster)  [unwired: 12 out]
                n289 = case shown="\"8-Contact Sample Hall\"" w390 {
                  tunnel: w391 -> [w394 w397 w415 w416 w434 w435 w452 w453]
                  frame "Van Der Pauw", Default {
                    # "Van Der Pauw test done so run Hall Effect test now"
                    n290 = call "Run Hall Effect Test.vi"("error in (no error)"=w394) -> ("error out"=w395:errorcluster)  [unwired: 10 out]
                    n291 = call <vilib>:"Simple Error Handler.vi"("error in (no error)"=w395) -> ()  [unwired: 1 in, 8 out]
                    n292 = local write "Test Progress"(u8 50 ("Test Progress")) -> ()
                  }
                  frame "Hall Effect" {
                    # "All tests complete.  Re-enable/disable buttons"
                    n293 = flat-sequence {
                      tunnel: w397 -> [w398]
                      frame #0 {
                        w399 = u8 0 ("Disabled")
                        n294 = property on="cmdClearData" class="Bool"(error in=w398, "Disabled"=w399) -> (error out=w400:errorcluster)  [unwired: 1 in, 1 out]
                        n295 = property on="cmdStart" class="Bool"(error in=w400, "Disabled"=w399) -> (error out=w406:errorcluster)  [unwired: 1 in, 1 out]
                        n296 = property on="cmdStop" class="Bool"(error in=w406, "Disabled"=u8 2) -> (error out=w405:errorcluster)  [unwired: 1 in, 1 out]
                        n297 = property on="Tab Control" class="TabCtl (strict)"(error in=w405) -> (error out=w401:errorcluster, "Pages"=w404:refnum<vi>[])  [unwired: 1 in, 1 out]
                        n298 = call "Tab Controls Disabled.vi"("Page"=0, "Disabled"=u8 0, "Tab Control Pages"=w404) -> ()  [unwired: 9 out]
                        n299 = call <vilib>:"Simple Error Handler.vi"("error in (no error)"=w401) -> ()  [unwired: 1 in, 8 out]
                      }
                      frame #1 {
                        n300 = local read "Status"() -> (w409:string)
                        n301 = local write "Test In Progress"(FALSE ("Test In Progress")) -> ()
                        n302 = Concatenate Strings(w409, "Idle.\r\n" ("string")) -> (w410:string)
                        n303 = local write "Test Progress"(u8 100 ("Test Progress")) -> ()
                        n304 = local write "Status"(w410) -> ()
                      }
                    }
                  }
                  frame "Bar Sample Resistivity" {
                    n305 = call "Run Hall of Bar Sample Test.vi"("error in (no error)"=w415) -> ("error out"=w414:errorcluster)  [unwired: 10 in]
                    n306 = call <vilib>:"Simple Error Handler.vi"("error in (no error)"=w414) -> ()  [unwired: 1 in, 8 out]
                    n307 = local write "Test Progress"(50) -> ()
                  }
                  frame "Bar Sample Hall " {
                    # "All tests complete.  Re-enable/disable buttons"
                    n308 = flat-sequence {
                      tunnel: w416 -> [w426]
                      frame #0 {
                        w422 = 0
                        n309 = property on="cmdClearData" class="Bool"(error in=w426, "DisabledEnum"=w422) -> (error out=w425:errorcluster)  [unwired: 1 in, 1 out]
                        n310 = property on="cmdStart" class="Bool"(error in=w425, "DisabledEnum"=w422) -> (error out=w424:errorcluster)  [unwired: 1 in, 1 out]
                        n311 = property on="cmdStop" class="Bool"(error in=w424, "DisabledEnum"=2) -> (error out=w423:errorcluster)  [unwired: 1 in, 1 out]
                        n312 = property on="Tab Control" class="TabCtl (strict)"(error in=w423) -> (error out=w417:errorcluster, "Pages"=w420:refnum<vi>[])  [unwired: 1 in, 1 out]
                        n313 = call "Tab Controls Disabled.vi"("Page"=0, "Disabled"=0, "Tab Control Pages"=w420) -> ()  [unwired: 9 out]
                        n314 = call <vilib>:"Simple Error Handler.vi"("error in (no error)"=w417) -> ()  [unwired: 1 in, 8 out]
                      }
                      frame #1 {
                        n315 = local read "Status"() -> (w428:string)
                        n316 = local write "Test In Progress"(FALSE ("Test In Progress")) -> ()
                        n317 = Concatenate Strings(w428, "Idle.\r\n" ("string")) -> (w429:string)
                        n318 = local write "Test Progress"(u8 100 ("Test Progress")) -> ()
                        n319 = local write "Status"(w429) -> ()
                      }
                    }
                  }
                  frame "6-Contact Sample Resistivity" {
                    n320 = call "Run Hall of 6-Contact Sample.vi"("error in (no error)"=w434) -> ("error out"=w433:errorcluster)  [unwired: 10 in]
                    n321 = call <vilib>:"Simple Error Handler.vi"("error in (no error)"=w433) -> ()  [unwired: 1 in, 8 out]
                    n322 = local write "Test Progress"(u8 50 ("Test Progress")) -> ()
                  }
                  frame "6-Contact Sample Hall" {
                    # "All tests complete.  Re-enable/disable buttons"
                    n323 = flat-sequence {
                      tunnel: w435 -> [w444]
                      frame #0 {
                        w437 = 0
                        w440 = 0
                        n324 = property on="cmdClearData" class="Bool"(error in=w444, "DisabledEnum"=w440) -> (error out=w443:errorcluster)  [unwired: 1 in, 1 out]
                        n325 = property on="cmdStart" class="Bool"(error in=w443, "DisabledEnum"=w440) -> (error out=w442:errorcluster)  [unwired: 1 in, 1 out]
                        n326 = property on="cmdStop" class="Bool"(error in=w442, "DisabledEnum"=2) -> (error out=w441:errorcluster)  [unwired: 1 in, 1 out]
                        n327 = property on="Tab Control" class="TabCtl (strict)"(error in=w441) -> (error out=w436:errorcluster, "Pages"=w438:refnum<vi>[])  [unwired: 1 in, 1 out]
                        n328 = call "Tab Controls Disabled.vi"("Page"=w437, "Disabled"=w437, "Tab Control Pages"=w438) -> ()  [unwired: 9 out]
                        n329 = call <vilib>:"Simple Error Handler.vi"("error in (no error)"=w436) -> ()  [unwired: 1 in, 8 out]
                      }
                      frame #1 {
                        n330 = local read "Status"() -> (w446:string)
                        n331 = local write "Test In Progress"(FALSE) -> ()
                        n332 = Concatenate Strings(w446, "Idle.\r\n" ("string")) -> (w447:string)
                        n333 = local write "Test Progress"(100) -> ()
                        n334 = local write "Status"(w447) -> ()
                      }
                    }
                  }
                  frame "8-Contact Sample Resistivity" {
                    n335 = call "Run Hall of 8-Contact Sample.vi"("error in (no error)"=w452) -> ("error out"=w451:errorcluster)  [unwired: 10 in]
                    n336 = call <vilib>:"Simple Error Handler.vi"("error in (no error)"=w451) -> ()  [unwired: 1 in, 8 out]
                    n337 = local write "Test Progress"(u8 50 ("Test Progress")) -> ()
                  }
                  frame "8-Contact Sample Hall" {
                    # "All tests complete.  Re-enable/disable buttons"
                    n338 = flat-sequence {
                      tunnel: w453 -> [w462]
                      frame #0 {
                        w455 = 0
                        w459 = 0
                        n339 = property on="cmdClearData" class="Bool"(error in=w462, "DisabledEnum"=w459) -> (error out=w461:errorcluster)  [unwired: 1 in, 1 out]
                        n340 = property on="cmdStart" class="Bool"(error in=w461, "DisabledEnum"=w459) -> (error out=w460:errorcluster)  [unwired: 1 in, 1 out]
                        n341 = property on="cmdStop" class="Bool"(error in=w460, "DisabledEnum"=2) -> (error out=w457:errorcluster)  [unwired: 1 in, 1 out]
                        n342 = property on="Tab Control" class="TabCtl (strict)"(error in=w457) -> (error out=w454:errorcluster, "Pages"=w456:refnum<vi>[])  [unwired: 1 in, 1 out]
                        n343 = call "Tab Controls Disabled.vi"("Page"=w455, "Disabled"=w455, "Tab Control Pages"=w456) -> ()  [unwired: 9 out]
                        n344 = call <vilib>:"Simple Error Handler.vi"("error in (no error)"=w454) -> ()  [unwired: 1 in, 8 out]
                      }
                      frame #1 {
                        n345 = local read "Status"() -> (w465:string)
                        n346 = local write "Test In Progress"(FALSE) -> ()
                        n347 = local write "Test Progress"(100) -> ()
                        n348 = Concatenate Strings(w465, "Idle.\r\n" ("string")) -> (w464:string)
                        n349 = local write "Status"(w464) -> ()
                      }
                    }
                  }
                }
              }
              frame "Test End User Abort", "Test End Error" {
                n350 = call-poly "Decode Message Data.vi"("Message Data"=w469, "error in"=w470) -> ("Error"=w468:errorcluster)  [unwired: 13 out]
                n351 = flat-sequence {
                  tunnel: w468 -> [w483]
                  frame #0 {
                    w471 = u8 0 ("Disabled")
                    # "An error occured and the test had to end.  Display\nthe error message then re-enable/disable controls"
                    n352 = call <vilib>:"Simple Error Handler.vi"("error in (no error)"=w483) -> ("error out"=w484:errorcluster, "message"=w475:string)  [unwired: 1 in, 6 out]
                    n353 = call <vilib>:"Clear Errors.vi"("error in (no error)"=w484) -> ("error out"=w477:errorcluster)  [unwired: 1 in, 5 out]
                    n354 = Concatenate Strings(w475, "\r\n") -> (w474:string)
                    n355 = control-ref of="Status"() -> (w478:refnum<vi>)
                    n356 = call "Append Status Message.vi"("Str Refnum"=w478, "Message"=w474, "error in (no error)"=w477) -> ("error out"=w472:errorcluster)  [unwired: 12 out]
                    n357 = property on="cmdClearData" class="Bool"(error in=w472, "Disabled"=w471) -> (error out=w473:errorcluster)  [unwired: 1 in, 1 out]
                    n358 = property on="cmdStart" class="Bool"(error in=w473, "Disabled"=w471) -> (error out=w485:errorcluster)  [unwired: 1 in, 1 out]
                    n359 = property on="cmdStop" class="Bool"(error in=w485, "Disabled"=u8 2) -> (error out=w482:errorcluster)  [unwired: 1 in, 1 out]
                    n360 = property on="Tab Control" class="TabCtl (strict)"(error in=w482) -> ("Pages"=w481:refnum<vi>[])  [unwired: 1 in, 2 out]
                    n361 = call "Tab Controls Disabled.vi"("Page"=0, "Disabled"=u8 0, "Tab Control Pages"=w481) -> ()  [unwired: 9 out]
                  }
                  frame #1 {
                    n362 = local write "Test In Progress"(FALSE ("Test In Progress")) -> ()
                    n363 = local write "Test Progress"(u8 0 ("Test Progress")) -> ()
                  }
                }
              }
            }
          }
          frame "mnuFileExit" {
            n364 = local read "Test In Progress"() -> (w490:bool)
            n365 = case shown="True" w490 {
              selector: w490 -> [w501 _]
              tunnel: [w501 w502] -> w489
              frame False {
              }
              frame True {
                n366 = Two Button Dialog(message="Test is still in progress.\n\nAre you sure you\nwant to quit?", 1:"No" ("F button name (\"Cancel\")"), 2:"Yes" ("T button name (\"OK\")")) -> (T button?=w502:bool)
              }
            }
            n367 = case shown="False" w489 {
              frame False {
                n368 = local read "Front Panel Window Default Size"() -> (w491:T1)
                n369 = local read "Programable Event"() -> (w493:refnum<user-event>)
                n370 = control-ref of="This VI"() -> (w492:refnum<vi>)
                n371 = property class="VI"(reference=w492, "Minimum Panel Size"=w491) -> ()  [unwired: 1 in, 2 out]
                n372 = Generate User Event(user event=w493, event data cluster=cluster{string} {"QUIT"} ("event data")) -> ()  [unwired: 2 in, 2 out]
              }
              frame True {
                n373 = local read "Front Panel Window Default Size"() -> (w495:T1)
                n374 = call "Abort Running Test.vi"() -> ("error out"=w498:errorcluster)  [unwired: 1 in, 10 out]
                n375 = call "Close Library.vi"("error in (no error)"=w498) -> ("error out"=w497:errorcluster)  [unwired: 10 out]
                n376 = local read "Programable Event"() -> (w499:refnum<user-event>)
                n377 = control-ref of="This VI"() -> (w496:refnum<vi>)
                n378 = property class="VI"(reference=w496, "Minimum Panel Size"=w495) -> ()  [unwired: 1 in, 2 out]
                n379 = Generate User Event(user event=w499, event data cluster=cluster{string} {"QUIT"} ("event data"), error in=w497) -> ()  [unwired: 1 in, 2 out]
              }
            }
          }
          frame "mnuFileLoad" {
            n380 = call "dlgLoadSettings"("prompt"="Save Test Parameters", "button label"="Save", "default name"="Test Paramters.xml", "pattern (all files)"="*.xml", "pattern label"="XML Test Parameters Files") -> ("selected path"=w507:path, "cancelled"=w508:bool, "error out"=w506:errorcluster)  [unwired: 2 in, 6 out]
            n381 = case shown="False" w508 {
              tunnel: w507 -> [w522 _]
              tunnel: w506 -> [w529 _]
              frame False {
                n382 = Open/Create/Replace File(file path (use dialog)=w522, error in=w529, operation (0:open)=T25."open", access (0:read/write)=enum16{"read/write", "read-only", "write-only"}."read-only") -> (refnum out=w524:refnum<file>, error out=w528:errorcluster)  [unwired: 3 out]
                n383 = Read from Text File(file (use dialog)=w524, count=-1, error in=w528) -> (refnum out=w526:refnum<file>, text=w525:string, error out=w527:errorcluster)  [unwired: 2 out]
                n384 = Close File(refnum=w526, error in=w527) -> (error out=w519:errorcluster)  [unwired: 1 out]
                n385 = Unflatten From XML(xml string=w525, type=T24 {"Test Identification"={"Sample Name"="", "User Name"=""}, "Test Input Parameters"={"Current Level "=1e-08, "Compliance Level"=7.0, "Soak Time"=0.0, "NPLC Voltmeter"=1.0, "Count Voltmeter"=2, "NPLC Ammeter"=0.57, "Count Ammeter"=1, "Sample Resistivity"=enum."High", "Sample Thickness"=10.0, "Magnetic Flux"=23.0, "Units"=enum."T", "Sample Dimensions x"=3.0, "Sample Dimensions y"=4.0, "Sample Dimensions D1"=5.0, "Sample Dimensions D2"=8.0, "Sample Width Ws"=6.0, "Slot Number of 3765 Card"=6}, "Test Type"={"Test Type"=enum."Bar Sample Resistivity and Hall Voltage Measurement"}} ("Test Paramters"), error in (no error)=w519) -> (value=w518:T24)  [unwired: 1 out]
                n386 = Unbundle By Name(w518) -> ("Test Identification"=w517:T12, "Test Input Parameters"=w515:T14, "Test Type"=w514:T11)
                n387 = local write "Test Input Parameters"(w515) -> ()
                n388 = local write "Test Identification"(w517) -> ()
                n389 = local write "Test Type"(w514) -> ()
              }
              frame True {
              }
            }
          }
          frame "mnuFileSave" {
            n390 = while {
              shift-right: [w536] -> _
              shift-left: _ -> [w544]
              shift-right: [w531] -> _
              shift-left: path "Test Paramters.xml" ("selected path") -> [w535]
              stop <- w542 stop-if-true
              n391 = Strip Path(path=w535) -> (stripped path=w534:path, name=w533:string)
              n392 = call "dlgSaveSettings"("start path"=w534, "prompt"="Save Test Parameters", "button label"="Save", "default name"=w533, "error in"=w544, "pattern (all files)"="*.xml", "pattern label"="XML Test Parameters Files") -> ("selected path"=w532:path, "cancelled"=w545:bool, "error out"=w543:errorcluster)  [unwired: 6 out]
              n393 = case shown="False" w545 {
                selector: w545 -> [_ w569]
                tunnel: w543 -> [w557 w570]
                tunnel: [w556 w570] -> w538
                tunnel: [w555 w569] -> w542
                tunnel: w532 -> [w553 w568]
                tunnel: [w552 w568] -> w531
                frame False {
                  n394 = local read "Test Identification"() -> (w564:T12)
                  n395 = Open/Create/Replace File(file path (use dialog)=w553, error in=w557, operation (0:open)=T25."replace or create with confirmation", access (0:read/write)=enum16{"read/write", "read-only", "write-only"}."write-only") -> (refnum out=w558:refnum<file>, cancelled=w554:bool, error out=w559:errorcluster)  [unwired: 2 out]
                  n396 = local read "Test Input Parameters"() -> (w563:T14)
                  n397 = local read "Test Type"() -> (w550:T11)
                  n398 = Bundle(cluster=T24 {"Test Identification"={"Sample Name"="", "User Name"=""}, "Test Input Parameters"={"Current Level "=1e-08, "Compliance Level"=7.0, "Soak Time"=0.0, "NPLC Voltmeter"=1.0, "Count Voltmeter"=2, "NPLC Ammeter"=0.57, "Count Ammeter"=1, "Sample Resistivity"=enum."High", "Sample Thickness"=10.0, "Magnetic Flux"=23.0, "Units"=enum."T", "Sample Dimensions x"=3.0, "Sample Dimensions y"=4.0, "Sample Dimensions D1"=5.0, "Sample Dimensions D2"=8.0, "Sample Width Ws"=6.0, "Slot Number of 3765 Card"=6}, "Test Type"={"Test Type"=enum."6-Contact Sample Resistivity and Hall Voltage Measurement"}} ("Test Paramters"), "Test Identification"=w564, "Test Input Parameters"=w563, "Test Type"=w550) -> (w565:T24)
                  n399 = Flatten To XML(anything=w565) -> (xml string=w562:string)
                  n400 = Not(x=w554) -> (.not. x?=w555:bool)
                  n401 = Write to Text File(file (use dialog)=w558, text=w562, error in=w559) -> (refnum out=w561:refnum<file>, error out=w560:errorcluster)  [unwired: 2 out]
                  n402 = Close File(refnum=w561, error in=w560) -> (path=w552:path, error out=w556:errorcluster)
                }
                frame True {
                }
              }
              n403 = Unbundle By Name(w538) -> ("code"=w541:i32)
              n404 = Equal?(x=w541, y=43) -> (x = y?=w539:bool)
              n405 = Select(t=errorcluster {"status"=FALSE, "code"=0, "source"=""}, s=w539, f=w538) -> (s? t:f=w536:errorcluster)
            }
          }
          frame "mnuInstrConfig" {
            n406 = local read "Instrument Locations"() -> (w574:T2)
            n407 = local read "Instruments"() -> (w575:T8)
            n408 = call "KHETS - Config Instruments.vi"("Instrument Locations In"=w574, "Instruments In"=w575) -> ("Instrument Locations Out"=w571:T2, "Clicked OK?"=w573:bool, "Instruments Out"=w572:T8)  [unwired: 7 out]
            n409 = local write "Instrument Locations"(w571) -> ()
            n410 = local write "Instruments"(w572) -> ()
            n411 = case shown="True" w573 {
              tunnel: w572 -> [_ w578]
              tunnel: w571 -> [_ w577]
              frame False {
              }
              frame True {
                # "If the config was changed,\nbe sure to save it to disk."
                n412 = call "KHE - Save Settings.vi"("Instrument Locations"=w577, "Instruments"=w578) -> ("error out"=w576:errorcluster)  [unwired: 1 in, 8 out]
                n413 = call <vilib>:"Simple Error Handler.vi"("error in (no error)"=w576) -> ()  [unwired: 1 in, 8 out]
              }
            }
          }
          frame "mnuInstrTest" {
            # "Instr. Loc. &\nTest Instr. Comm."
            n414 = control-ref of="Status"() -> (w593:refnum<vi>)
            n415 = local read "Instruments"() -> (w585:T8)
            n416 = local read "Instrument Locations"() -> (w606:T2)
            n417 = call "Append Status Message.vi"("Str Refnum"=w593, "Message"="Testing communications..." ("string")) -> ("error out"=w594:errorcluster)  [unwired: 1 in, 12 out]
            n418 = property on="Tab Control" class="TabCtl (strict)"(error in=w594) -> (error out=w602:errorcluster, "Pages"=w605:refnum<vi>[])  [unwired: 1 in, 1 out]
            n419 = Unbundle By Name(w585) -> ("Ammeter"=w584:T4, "Current Source"=w583:T5, "Switch"=w582:T6, "Voltmeter"=w581:T7)
            n420 = call "Tab Controls Disabled.vi"("Page"=0, "Disabled"=u8 2, "Tab Control Pages"=w605) -> ()  [unwired: 9 out]
            n421 = Unbundle By Name(w606) -> ("Voltmeter Location"=w589:refnum<visa-resource-name>, "Switch Location"=w590:refnum<visa-resource-name>, "Ammeter Location"=w587:refnum<visa-resource-name>, "Current Source Location"=w586:refnum<visa-resource-name>)
            n422 = property on="cmdStart" class="Bool"(error in=w602, "Disabled"=u8 2) -> (error out=w579:errorcluster, "Disabled"=w600:u8)  [unwired: 1 in, 1 out]
            n423 = call "Configure Instruments.vi"("Ammeter"=w584, "error in (no error)"=w579, "Voltmeter"=w581, "Switch"=w582, "Current Source"=w583) -> ("error out"=w580:errorcluster)  [unwired: 6 in]
            n424 = call "Configure Instrument Locations.vi"("V-Meter"=w589, "Switch"=w590, "error in (no error)"=w580, "I-SRC"=w586, "Ammeter"=w587) -> ("error out"=w591:errorcluster)  [unwired: 1 in, 5 out]
            n425 = call "Test Instrument Communications.vi"("error in (no error)"=w591) -> ("error out"=w588:errorcluster)  [unwired: 10 out]
            n426 = case shown="No Error" w588 {
              selector: w588 -> [w610 w622]
              tunnel: [w611 w620] -> w603
              frame No Error {
                n427 = control-ref of="Status"() -> (w612:refnum<vi>)
                n428 = call "Append Status Message.vi"("Str Refnum"=w612, "Message"="Done\r\n" ("string"), "error in (no error)"=w610) -> ("error out"=w611:errorcluster)  [unwired: 12 out]
                n429 = One Button Dialog(message="Communications test passed.") -> ()  [unwired: 2 out]
              }
              frame Error {
                n430 = control-ref of="Status"() -> (w619:refnum<vi>)
                n431 = call <vilib>:"Simple Error Handler.vi"("error in (no error)"=w622) -> ("error out"=w621:errorcluster, "message"=w616:string)  [unwired: 1 in, 6 out]
                n432 = Concatenate Strings("Error!\r\n" ("string"), w616, "\r\n") -> (w618:string)
                n433 = call <vilib>:"Clear Errors.vi"("error in (no error)"=w621) -> ("error out"=w620:errorcluster)  [unwired: 1 in, 5 out]
                n434 = call "Append Status Message.vi"("Str Refnum"=w619, "Message"=w618) -> ()  [unwired: 1 in, 13 out]
              }
            }
            n435 = property on="cmdStart" class="Bool"(error in=w603, "Disabled"=w600) -> (error out=w596:errorcluster)  [unwired: 1 in, 1 out]
            n436 = property on="Tab Control" class="TabCtl (strict)"(error in=w596) -> (error out=w607:errorcluster, "Pages"=w595:refnum<vi>[])  [unwired: 1 in, 1 out]
            n437 = call "Tab Controls Disabled.vi"("Page"=0, "Disabled"=u8 0, "Tab Control Pages"=w595) -> ()  [unwired: 9 out]
            n438 = control-ref of="Status"() -> (w609:refnum<vi>)
            n439 = call "Append Status Message.vi"("Str Refnum"=w609, "Message"="Idle.\r\n" ("string"), "error in (no error)"=w607) -> ()  [unwired: 13 out]
          }
          frame "mnuInstrCur_Val" {
            # "Save the 648x Measured Currents"
            n440 = call "Show_Test_Currents.vi"() -> ()  [unwired: 1 in]
          }
          frame "mnuHelpAbout" {
            n441 = call "KHETS - About.vi"() -> ()  [unwired: 1 in]
          }
          frame Default {
          }
        }
      }
      frame Error {
        n442 = property class="App"() -> ("App.Kind"=w625:T26)  [unwired: 2 in, 2 out]
        n443 = Equal?(x=w625, y=T26."Run Time System") -> (x = y?=w623:bool)
        n444 = Quit LabVIEW(quit? (T)=w623) -> ()
      }
    }
  }
  n445 = while {
    shift-right: [w629] -> w18
    shift-left: w14 -> [w632]
    tunnel: w2 -> [w633]
    tunnel: w10 -> [w627]
    tunnel: [w626] -> w13
    stop <- w630 stop-if-true
    n446 = event shown="[8] Menu Selection (User)" {
      selector: w627 -> [_ _ _ _ _ _ _ _ _]
      dyn-events: [_ _ _ _ _ _ _ _ _] -> w626
      timeout: _ -> [_ _ _ _ _ _ _ _ _]
      tunnel: w633 -> [w637 w639 w642 w646 w650 w655 w660 w671 w674]
      tunnel: w632 -> [w636 w640 w643 w647 w652 w656 w661 w672 w676]
      tunnel: [w635 w641 w644 w648 w653 w657 w662 w670 w675] -> w629
      tunnel: [_ _ _ _ _ _ w658 _ _] -> w631
      event "cmdStart": Value Change {
        n447 = event-data() -> ()  [unwired: 2 out]
        n448 = Enqueue Element(queue=w637, element="cmdStart_Click", error in (no error)=w636) -> (error out=w635:errorcluster)  [unwired: 3 out]
      }
      event "cmdStop": Value Change {
        n449 = event-data() -> ()  [unwired: 2 out]
        n450 = Enqueue Element(queue=w639, element="cmdStop_Click", error in (no error)=w640) -> (error out=w641:errorcluster)  [unwired: 3 out]
      }
      event "cmdClearData": Value Change {
        n451 = event-data() -> ()  [unwired: 2 out]
        n452 = Enqueue Element(queue=w642, element="cmdClearData_Click", error in (no error)=w643) -> (error out=w644:errorcluster)  [unwired: 3 out]
      }
      event "cmdSaveData": Value Change {
        n453 = event-data() -> ()  [unwired: 2 out]
        n454 = Enqueue Element(queue=w646, element="cmdSaveData_Click", error in (no error)=w647) -> (error out=w648:errorcluster)  [unwired: 3 out]
      }
      event "cmdIndex": Value Change {
        n455 = event-data() -> ()  [unwired: 2 out]
        n456 = Enqueue Element(queue=w650, element="cmdIndex_Click", error in (no error)=w652) -> (error out=w653:errorcluster)  [unwired: 3 out]
      }
      event "cmdBack": Value Change {
        n457 = event-data() -> ()  [unwired: 2 out]
        n458 = Enqueue Element(queue=w655, element="cmdBack_Click", error in (no error)=w656) -> (error out=w657:errorcluster)  [unwired: 3 out]
      }
      event User Event {
        n459 = event-data() -> ("Event Name"=w659:string)  [unwired: 1 out]
        n460 = Equal?(x="QUIT", y=w659) -> (x = y?=w658:bool)
        n461 = case shown="False" w658 {
          tunnel: [w667 w668] -> w662
          tunnel: w661 -> [w666 w668]
          tunnel: w660 -> [w665 _]
          tunnel: w659 -> [w664 _]
          frame False {
            n462 = Enqueue Element(queue=w665, element=w664, error in (no error)=w666) -> (error out=w667:errorcluster)  [unwired: 3 out]
          }
          frame True {
          }
        }
      }
      event User Event {
        n463 = event-data() -> ("Event Name"=w669:string)  [unwired: 1 out]
        n464 = Enqueue Element(queue=w671, element=w669, error in (no error)=w672) -> (error out=w670:errorcluster)  [unwired: 3 out]
      }
      event Menu Selection (User) {
        n465 = event-data() -> ("ItemTag"=w673:string)  [unwired: 1 out]
        n466 = Enqueue Element(queue=w674, element=w673, error in (no error)=w676) -> (error out=w675:errorcluster)  [unwired: 3 out]
      }
    }
    n467 = Unbundle By Name(w629) -> ("status"=w628:bool)
    n468 = Or(x=w628, y=w631) -> (x .or. y?=w630:bool)
  }
  n469 = Release Queue(queue=w2, error in (no error)=w18) -> (error out=w12:errorcluster)  [unwired: 3 out]
  n470 = Unregister For Events(event registration refnum=w13, error in=w12) -> (error out=w11:errorcluster)
  n471 = Destroy User Event(user event=w4, error in=w11) -> (error out=w1:errorcluster)
  n472 = call "Close Library.vi"("error in (no error)"=w1) -> ()  [unwired: 11 out]
